vi "_LoadParameterTable.vi"(6 "ScanMode":string="Q1Pos") -> (0 "error out":errorcluster, 2 "ParameterList":string[][](array[string])=[["Q1 RF", "1", "10", "2150", "400", "0", "218.45", "64", "Quadrupole 1 RF", "\n      ", "\n      "], ["Q1 DC", "4", "10", "2150", "600", "0", "218.45", "64", "Quadrupole 1 DC", "\n      ", "\n      "], ["Q1 RR", "7", "0", "64000", "32768", "32768", "1", "64", "Quadrupole 1 PW", "\n      ", "\n      "], ["Q2 RF", "2", "10", "2150", "400", "0", "218.45", "64", "Quadrupole 2 RF", "\n      ", "\n      "], ["Q2 DC", "5", "10", "2150", "600", "0", "218.45", "64", "Quadrupole 2 DC", "\n      ", "\n      "], ["Q2 RR", "9", "0", "64000", "32768", "32768", "1", "64", "Quadrupole 2 PW", "\n      ", "\n      "], ["M1 RF", "3", "0", "600", "500", "0", "14.7", "6", "Multipole 1 RF", "Fixed", "Operator"], ["EV", "20", "0", "200", "100", "32768", "-65.7", "7", "Entrance Voltage", "Operator", "Operator"], ["ED", "21", "0", "200", "90", "32768", "-65.5", "7", "Entrance Deflector", "Operator", "Operator"], ["M1", "19", "-10", "5", "-1", "32768", "-65.6", "7", "Multipole 1", "Equation", "Equation"], ["L1", "18", "-10", "5", "-2", "32760", "-65.9", "7", "Multipole Lens 1", "Equation", "Equation"], ["M2", "22", "-10", "5", "-3", "32768", "-66", "7", "Multipole 2", "Fixed", "Fixed"], ["L2", "11", "-10", "5", "-4", "32768", "-65.9", "7", "Multipole Lens 2", "Equation", "Equation"], ["PF", "12", "-50", "5", "-15", "32768", "-65.8", "7", "Prefilter 1", "Equation", "Operator"], ["Q1", "6", "-10", "0", "-4.5", "32755", "-131.3", "11", "Quadrupole 1", "Equation", "Equation"], ["CC L1", "13", "-100", "10", "-10", "32768", "-65.8", "7", "Collision Cell Lens 1", "Equation", "Operator"], ["CC L2", "14", "-400", "0", "-120", "32768", "-65.8", "7", "Collision Cell Lens 2", "Fixed", "Operator"], ["CC", "23", "-150", "0", "-50", "32768", "-65.8", "7", "Collision Energy", "Fixed", "Fixed"], ["CC AF", "10", "0", "400", "100", "32768", "-65.8", "7", "Axial Field", "Fixed", "Fixed"], ["CC L3", "15", "-400", "0", "-51", "32768", "-65.7", "7", "Collision Cell Lens 3", "Equation", "Operator"], ["CC L4", "16", "-400", "0", "-62", "32768", "-65.7", "7", "Collision Cell Lens 4", "Equation", "Operator"], ["Q2", "8", "-150", "0", "-52", "32756", "-131.3", "11", "Quadrupole 2", "Equation", "Equation"], ["ID", "17", "-400", "0", "-90", "32768", "-65.8", "7", "Detector Deflector", "Equation", "Equation"], ["DISC", "32", "10", "2000", "15", "-5", "1.23", "18", "Discriminator", "Fixed", "Fixed"], ["DV", "34", "1600", "3500", "2000", "0", "0.415", "18", "Detector Voltage", "Operator", "Operator"], ["DET horn", "200", "0", "5500", "5500", "0", "0.415", "16", "Detector Horn", "Fixed", "Fixed"], ["LS400A", "36", "0", "420", "420", "0", "8.4", "64", "Lens Power Supply A +400", "\n      ", "\n      "], ["LS-400A", "37", "-420", "-55", "-420", "-433", "-8.4", "64", "Lens Power Supply A -400", "\n      ", "\n      "], ["LS400B", "38", "0", "420", "420", "0", "8.4", "64", "Lens Power Supply B +400", "\n      ", "\n      "], ["LS-400B", "39", "-420", "-55", "-420", "-433", "-8.4", "64", "Lens Power Supply B  -400", "\n      ", "\n      "], ["QPS800", "40", "110", "600", "600", "0", "4.25", "64", "Quad Power Supply +800", "\n      ", "\n      "], ["QPS-800", "41", "-110", "-110", "-600", "-433", "-4.2", "64", "Quad Power Supply -800", "\n      ", "\n      "], ["DG", "26", "50", "300", "80", "0", "32.765", "32", "Drying Gas", "Operator", "Operator"], ["NG1", "27", "0", "450", "0", "0", "32.765", "32", "Nebulizer Gas 1", "Operator", "Operator"], ["HG1", "29", "0", "350", "0", "0", "32.765", "32", "Heating Gas 1", "Equation", "Equation"], ["NG2", "28", "0", "450", "0", "0", "32.765", "32", "Nebulizer Gas 2", "Operator", "Operator"], ["HG2", "30", "0", "350", "0", "0", "32.765", "32", "Heating Gas 2", "Equation", "Equation"], ["CC P", "43", "0", "500", "0", "0", "32.765", "6", "Collision Pressure", "Fixed", "Fixed"], ["SX", "42", "0", "500", "500", "0", "32.765", "32", "Source Exhaust", "Fixed", "Fixed"], ["ISV2", "204", "0", "5850", "0", "0", "0.0436", "34", "ElectroSpray V2", "Operator", "Operator"], ["ISV1", "203", "0", "5850", "0", "0", "0.0436", "34", "ElectroSpray V1", "Operator", "Operator"], ["CD", "202", "0", "5", "0", "0", "51", "34", "Corona Discharge", "Operator", "Operator"], ["CAP", "201", "0", "1100", "1000", "0", "0.22", "34", "Curtain Cap", "Fixed", "Fixed"], ["HSID T", "81", "0", "320", "200", "0", "1", "32", "HSID Temperature", "Operator", "Operator"], ["P1 T", "86", "0", "500", "0", "0", "1", "32", "Source 1 Temp", "Operator", "Operator"], ["P2 T", "84", "0", "500", "0", "0", "1", "32", "Source 2 Temp", "Operator", "Operator"]])   [LabVIEW 2012]
uses:
  <vilib>/xml/Load XML File.vi
  <vilib>/xml/Close Reference(Node).vi
  <vilib>/xml/NI_XML.lvlib
  <resource>/objmgr/DOMUserDefRef.rc
panel:
  out "ScanType":string[](array[string])=["<ScanType name=\"Q1Positive\">\n    <ParaRow Row=\"1\">\n      <Parameter>Q1 RF</Parameter>\n      <Channal>1</Channal>\n      <UserMin>10</UserMin>\n      <UserMax>2150</UserMax>\n      <UserDefault>400</UserDefault>\n      <CalibrationOffset>0</CalibrationOffset>\n      <CalibrationSlope>218.45</CalibrationSlope>\n      <ParameterType>64</ParameterType>\n      <Description>Quadrupole 1 RF</Description>\n      <Linked>\n      </Linked>\n      <Unlinked>\n      </Unlinked>\n      <Location>\n      </Location>\n    </ParaRow>\n    <ParaRow Row=\"2\">\n      <Parameter>Q1 DC</Parameter>\n      <Channal>4</Channal>\n      <UserMin>10</UserMin>\n      <UserMax>2150</UserMax>\n      <UserDefault>600</UserDefault>\n      <CalibrationOffset>0</CalibrationOffset>\n      <CalibrationSlope>218.45</CalibrationSlope>\n      <ParameterType>64</ParameterType>\n      <Description>Quadrupole 1 DC</Description>\n      <Linked>\n      </Linked>\n      <Unlinked>\n      </Unlinked>\n      <Location>\n      </Location>\n    </ParaRow>\n    <ParaRow Row=\"3\">\n      <Parameter>Q1 RR</Parameter>\n      <Channal>7</Channal>\n      <UserMin>0</UserMin>\n      <UserMax>64000</UserMax>\n      <UserDefault>32768</UserDefault>\n      <CalibrationOffset>32768</CalibrationOffset>\n      <CalibrationSlope>1</CalibrationSlope>\n      <ParameterType>64</ParameterType>\n      <Description>Quadrupole 1 PW</Description>\n      <Linked>\n      </Linked>\n      <Unlinked>\n      </Unlinked>\n      <Location>\n      </Location>\n    </ParaRow>\n    <ParaRow Row=\"4\">\n      <Parameter>Q2 RF</Parameter>\n      <Channal>2</Channal>\n      <UserMin>10</UserMin>\n      <UserMax>2150</UserMax>\n      <UserDefault>400</UserDefault>\n      <CalibrationOffset>0</CalibrationOffset>\n      <CalibrationSlope>218.45</CalibrationSlope>\n      <ParameterType>64</ParameterType>\n      <Description>Quadrupole 2 RF</Description>\n      <Linked>\n      </Linked>\n      <Unlinked>\n      </Unlinked>\n      <Location>\n      </Location>\n    </ParaRow>\n    <ParaRow Row=\"5\">\n      <Parameter>Q2 DC</Parameter>\n      <Channal>5</Channal>\n      <UserMin>10</UserMin>\n      <UserMax>2150</UserMax>\n      <UserDefault>600</UserDefault>\n      <CalibrationOffset>0</CalibrationOffset>\n      <CalibrationSlope>218.45</CalibrationSlope>\n      <ParameterType>64</ParameterType>\n      <Description>Quadrupole 2 DC</Description>\n      <Linked>\n      </Linked>\n      <Unlinked>\n      </Unlinked>\n      <Location>\n      </Location>\n    </ParaRow>\n    <ParaRow Row=\"6\">\n      <Parameter>Q2 RR</Parameter>\n      <Channal>9</Channal>\n      <UserMin>0</UserMin>\n      <UserMax>64000</UserMax>\n      <UserDefault>32768</UserDefault>\n      <CalibrationOffset>32768</CalibrationOffset>\n      <CalibrationSlope>1</CalibrationSlope>\n      <ParameterType>64</ParameterType>\n      <Description>Quadrupole 2 PW</Description>\n      <Linked>\n      </Linked>\n      <Unlinked>\n      </Unlinked>\n      <Location>\n      </Location>\n    </ParaRow>\n    <ParaRow Row=\"7\">\n      <Parameter>M1 RF</Parameter>\n      <Channal>3</Channal>\n      <UserMin>0</UserMin>\n      <UserMax>600</UserMax>\n      <UserDefault>500</UserDefault>\n      <CalibrationOffset>0</CalibrationOffset>\n      <CalibrationSlope>14.7</CalibrationSlope>\n      <ParameterType>6</ParameterType>\n      <Description>Multipole 1 RF</Description>\n      <Linked>Fixed</Linked>\n      <Unlinked>Operator</Unlinked>\n      <Location>Compound</Location>\n    </ParaRow>\n    <ParaRow Row=\"8\">\n      <Parameter>EV</Parameter>\n      <Channal>20</Channal>\n      <UserMin>0</UserMin>\n      <UserMax>200</UserMax>\n      <UserDefault>100</UserDefault>\n      <CalibrationOffset>32768</CalibrationOffset>\n      <CalibrationSlope>-65.7</CalibrationSlope>\n      <ParameterType>7</ParameterType>\n      <Description>Entrance Voltage</Description>\n      <Linked>Operator</Linked>\n      <Unlinked>Operator</Unlinked>\n      <Location>Compound</Location>\n    </ParaRow>\n    <ParaRow Row=\"9\">\n      <Parameter>ED</Parameter>\n      <Channal>21</Channal>\n      <UserMin>0</UserMin>\n      <UserMax>200</UserMax>\n      <UserDefault>90</UserDefault>\n      <CalibrationOffset>32768</CalibrationOffset>\n      <CalibrationSlope>-65.5</CalibrationSlope>\n      <ParameterType>7</ParameterType>\n      <Description>Entrance Deflector</Description>\n      <Linked>Operator</Linked>\n      <Unlinked>Operator</Unlinked>\n      <Location>Compound</Location>\n    </ParaRow>\n    <ParaRow Row=\"10\">\n      <Parameter>M1</Parameter>\n      <Channal>19</Channal>\n      <UserMin>-10</UserMin>\n      <UserMax>5</UserMax>\n      <UserDefault>-1</UserDefault>\n      <CalibrationOffset>32768</CalibrationOffset>\n      <CalibrationSlope>-65.6</CalibrationSlope>\n      <ParameterType>7</ParameterType>\n      <Description>Multipole 1</Description>\n      <Linked>Equation</Linked>\n      <Unlinked>Equation</Unlinked>\n      <Location>Compound</Location>\n    </ParaRow>\n    <ParaRow Row=\"11\">\n      <Parameter>L1</Parameter>\n      <Channal>18</Channal>\n      <UserMin>-10</UserMin>\n      <UserMax>5</UserMax>\n      <UserDefault>-2</UserDefault>\n      <CalibrationOffset>32760</CalibrationOffset>\n      <CalibrationSlope>-65.9</CalibrationSlope>\n      <ParameterType>7</ParameterType>\n      <Description>Multipole Lens 1</Description>\n      <Linked>Equation</Linked>\n      <Unlinked>Equation</Unlinked>\n      <Location>Compound</Location>\n    </ParaRow>\n    <ParaRow Row=\"12\">\n      <Parameter>M2</Parameter>\n      <Channal>22</Channal>\n      <UserMin>-10</UserMin>\n      <UserMax>5</UserMax>\n      <UserDefault>-3</UserDefault>\n      <CalibrationOffset>32768</CalibrationOffset>\n      <CalibrationSlope>-66</CalibrationSlope>\n      <ParameterType>7</ParameterType>\n      <Description>Multipole 2</Description>\n      <Linked>Fixed</Linked>\n      <Unlinked>Fixed</Unlinked>\n      <Location>Compound</Location>\n    </ParaRow>\n    <ParaRow Row=\"13\">\n      <Parameter>L2</Parameter>\n      <Channal>11</Channal>\n      <UserMin>-10</UserMin>\n      <UserMax>5</UserMax>\n      <UserDefault>-4</UserDefault>\n      <CalibrationOffset>32768</CalibrationOffset>\n      <CalibrationSlope>-65.9</CalibrationSlope>\n      <ParameterType>7</ParameterType>\n      <Description>Multipole Lens 2</Description>\n      <Linked>Equation</Linked>\n      <Unlinked>Equation</Unlinked>\n      <Location>Compound</Location>\n    </ParaRow>\n    <ParaRow Row=\"14\">\n      <Parameter>PF</Parameter>\n      <Channal>12</Channal>\n      <UserMin>-50</UserMin>\n      <UserMax>5</UserMax>\n      <UserDefault>-15</UserDefault>\n      <CalibrationOffset>32768</CalibrationOffset>\n      <CalibrationSlope>-65.8</CalibrationSlope>\n      <ParameterType>7</ParameterType>\n      <Description>Prefilter 1</Description>\n      <Linked>Equation</Linked>\n      <Unlinked>Operator</Unlinked>\n      <Location>Compound</Location>\n    </ParaRow>\n    <ParaRow Row=\"15\">\n      <Parameter>Q1</Parameter>\n      <Channal>6</Channal>\n      <UserMin>-10</UserMin>\n      <UserMax>0</UserMax>\n      <UserDefault>-4.5</UserDefault>\n      <CalibrationOffset>32755</CalibrationOffset>\n      <CalibrationSlope>-131.3</CalibrationSlope>\n      <ParameterType>11</ParameterType>\n      <Description>Quadrupole 1</Description>\n      <Linked>Equation</Linked>\n      <Unlinked>Equation</Unlinked>\n      <Location>Resolution</Location>\n    </ParaRow>\n    <ParaRow Row=\"16\">\n      <Parameter>CC L1</Parameter>\n      <Channal>13</Channal>\n      <UserMin>-100</UserMin>\n      <UserMax>10</UserMax>\n      <UserDefault>-10</UserDefault>\n      <CalibrationOffset>32768</CalibrationOffset>\n      <CalibrationSlope>-65.8</CalibrationSlope>\n      <ParameterType>7</ParameterType>\n      <Description>Collision Cell Lens 1</Description>\n      <Linked>Equation</Linked>\n      <Unlinked>Operator</Unlinked>\n      <Location>Compound</Location>\n    </ParaRow>\n    <ParaRow Row=\"17\">\n      <Parameter>CC L2</Parameter>\n      <Channal>14</Channal>\n      <UserMin>-400</UserMin>\n      <UserMax>0</UserMax>\n      <UserDefault>-120</UserDefault>\n      <CalibrationOffset>32768</CalibrationOffset>\n      <CalibrationSlope>-65.8</CalibrationSlope>\n      <ParameterType>7</ParameterType>\n      <Description>Collision Cell Lens 2</Description>\n      <Linked>Fixed</Linked>\n      <Unlinked>Operator</Unlinked>\n      <Location>Compound</Location>\n    </ParaRow>\n    <ParaRow Row=\"18\">\n      <Parameter>CC</Parameter>\n      <Channal>23</Channal>\n      <UserMin>-150</UserMin>\n      <UserMax>0</UserMax>\n      <UserDefault>-50</UserDefault>\n      <CalibrationOffset>32768</CalibrationOffset>\n      <CalibrationSlope>-65.8</CalibrationSlope>\n      <ParameterType>7</ParameterType>\n      <Description>Collision Energy</Description>\n      <Linked>Fixed</Linked>\n      <Unlinked>Fixed</Unlinked>\n      <Location>Compound</Location>\n    </ParaRow>\n    <ParaRow Row=\"19\">\n      <Parameter>CC AF</Parameter>\n      <Channal>10</Channal>\n      <UserMin>0</UserMin>\n      <UserMax>400</UserMax>\n      <UserDefault>100</UserDefault>\n      <CalibrationOffset>32768</CalibrationOffset>\n      <CalibrationSlope>-65.8</CalibrationSlope>\n      <ParameterType>7</ParameterType>\n      <Description>Axial Field</Description>\n      <Linked>Fixed</Linked>\n      <Unlinked>Fixed</Unlinked>\n      <Location>Compound</Location>\n    </ParaRow>\n    <ParaRow Row=\"20\">\n      <Parameter>CC L3</Parameter>\n      <Channal>15</Channal>\n      <UserMin>-400</UserMin>\n      <UserMax>0</UserMax>\n      <UserDefault>-51</UserDefault>\n      <CalibrationOffset>32768</CalibrationOffset>\n      <CalibrationSlope>-65.7</CalibrationSlope>\n      <ParameterType>7</ParameterType>\n      <Description>Collision Cell Lens 3</Description>\n      <Linked>Equation</Linked>\n      <Unlinked>Operator</Unlinked>\n      <Location>Compound</Location>\n    </ParaRow>\n    <ParaRow Row=\"21\">\n      <Parameter>CC L4</Parameter>\n      <Channal>16</Channal>\n      <UserMin>-400</UserMin>\n      <UserMax>0</UserMax>\n      <UserDefault>-62</UserDefault>\n      <CalibrationOffset>32768</CalibrationOffset>\n      <CalibrationSlope>-65.7</CalibrationSlope>\n      <ParameterType>7</ParameterType>\n      <Description>Collision Cell Lens 4</Description>\n      <Linked>Equation</Linked>\n      <Unlinked>Operator</Unlinked>\n      <Location>Compound</Location>\n    </ParaRow>\n    <ParaRow Row=\"22\">\n      <Parameter>Q2</Parameter>\n      <Channal>8</Channal>\n      <UserMin>-150</UserMin>\n      <UserMax>0</UserMax>\n      <UserDefault>-52</UserDefault>\n      <CalibrationOffset>32756</CalibrationOffset>\n      <CalibrationSlope>-131.3</CalibrationSlope>\n      <ParameterType>11</ParameterType>\n      <Description>Quadrupole 2</Description>\n      <Linked>Equation</Linked>\n      <Unlinked>Equation</Unlinked>\n      <Location>Resolution</Location>\n    </ParaRow>\n    <ParaRow Row=\"23\">\n      <Parameter>ID</Parameter>\n      <Channal>17</Channal>\n      <UserMin>-400</UserMin>\n      <UserMax>0</UserMax>\n      <UserDefault>-90</UserDefault>\n      <CalibrationOffset>32768</CalibrationOffset>\n      <CalibrationSlope>-65.8</CalibrationSlope>\n      <ParameterType>7</ParameterType>\n      <Description>Detector Deflector</Description>\n      <Linked>Equation</Linked>\n      <Unlinked>Equation</Unlinked>\n      <Location>Compound</Location>\n    </ParaRow>\n    <ParaRow Row=\"24\">\n      <Parameter>DISC</Parameter>\n      <Channal>32</Channal>\n      <UserMin>10</UserMin>\n      <UserMax>2000</UserMax>\n      <UserDefault>15</UserDefault>\n      <CalibrationOffset>-5</CalibrationOffset>\n      <CalibrationSlope>1.23</CalibrationSlope>\n      <ParameterType>18</ParameterType>\n      <Description>Discriminator</Description>\n      <Linked>Fixed</Linked>\n      <Unlinked>Fixed</Unlinked>\n      <Location>Detector</Location>\n    </ParaRow>\n    <ParaRow Row=\"25\">\n      <Parameter>DV</Parameter>\n      <Channal>34</Channal>\n      <UserMin>1600</UserMin>\n      <UserMax>3500</UserMax>\n      <UserDefault>2000</UserDefault>\n      <CalibrationOffset>0</CalibrationOffset>\n      <CalibrationSlope>0.415</CalibrationSlope>\n      <ParameterType>18</ParameterType>\n      <Description>Detector Voltage</Description>\n      <Linked>Operator</Linked>\n      <Unlinked>Operator</Unlinked>\n      <Location>Detector</Location>\n    </ParaRow>\n    <ParaRow Row=\"26\">\n      <Parameter>DET horn</Parameter>\n      <Channal>200</Channal>\n      <UserMin>0</UserMin>\n      <UserMax>5500</UserMax>\n      <UserDefault>5500</UserDefault>\n      <CalibrationOffset>0</CalibrationOffset>\n      <CalibrationSlope>0.415</CalibrationSlope>\n      <ParameterType>16</ParameterType>\n      <Description>Detector Horn</Description>\n      <Linked>Fixed</Linked>\n      <Unlinked>Fixed</Unlinked>\n      <Location>Detector</Location>\n    </ParaRow>\n    <ParaRow Row=\"27\">\n      <Parameter>LS400A</Parameter>\n      <Channal>36</Channal>\n      <UserMin>0</UserMin>\n      <UserMax>420</UserMax>\n      <UserDefault>420</UserDefault>\n      <CalibrationOffset>0</CalibrationOffset>\n      <CalibrationSlope>8.4</CalibrationSlope>\n      <ParameterType>64</ParameterType>\n      <Description>Lens Power Supply A +400</Description>\n      <Linked>\n      </Linked>\n      <Unlinked>\n      </Unlinked>\n      <Location>\n      </Location>\n    </ParaRow>\n    <ParaRow Row=\"28\">\n      <Parameter>LS-400A</Parameter>\n      <Channal>37</Channal>\n      <UserMin>-420</UserMin>\n      <UserMax>-55</UserMax>\n      <UserDefault>-420</UserDefault>\n      <CalibrationOffset>-433</CalibrationOffset>\n      <CalibrationSlope>-8.4</CalibrationSlope>\n      <ParameterType>64</ParameterType>\n      <Description>Lens Power Supply A -400</Description>\n      <Linked>\n      </Linked>\n      <Unlinked>\n      </Unlinked>\n      <Location>\n      </Location>\n    </ParaRow>\n    <ParaRow Row=\"29\">\n      <Parameter>LS400B</Parameter>\n      <Channal>38</Channal>\n      <UserMin>0</UserMin>\n      <UserMax>420</UserMax>\n      <UserDefault>420</UserDefault>\n      <CalibrationOffset>0</CalibrationOffset>\n      <CalibrationSlope>8.4</CalibrationSlope>\n      <ParameterType>64</ParameterType>\n      <Description>Lens Power Supply B +400</Description>\n      <Linked>\n      </Linked>\n      <Unlinked>\n      </Unlinked>\n      <Location>\n      </Location>\n    </ParaRow>\n    <ParaRow Row=\"30\">\n      <Parameter>LS-400B</Parameter>\n      <Channal>39</Channal>\n      <UserMin>-420</UserMin>\n      <UserMax>-55</UserMax>\n      <UserDefault>-420</UserDefault>\n      <CalibrationOffset>-433</CalibrationOffset>\n      <CalibrationSlope>-8.4</CalibrationSlope>\n      <ParameterType>64</ParameterType>\n      <Description>Lens Power Supply B  -400</Description>\n      <Linked>\n      </Linked>\n      <Unlinked>\n      </Unlinked>\n      <Location>\n      </Location>\n    </ParaRow>\n    <ParaRow Row=\"31\">\n      <Parameter>QPS800</Parameter>\n      <Channal>40</Channal>\n      <UserMin>110</UserMin>\n      <UserMax>600</UserMax>\n      <UserDefault>600</UserDefault>\n      <CalibrationOffset>0</CalibrationOffset>\n      <CalibrationSlope>4.25</CalibrationSlope>\n      <ParameterType>64</ParameterType>\n      <Description>Quad Power Supply +800</Description>\n      <Linked>\n      </Linked>\n      <Unlinked>\n      </Unlinked>\n      <Location>\n      </Location>\n    </ParaRow>\n    <ParaRow Row=\"32\">\n      <Parameter>QPS-800</Parameter>\n      <Channal>41</Channal>\n      <UserMin>-110</UserMin>\n      <UserMax>-110</UserMax>\n      <UserDefault>-600</UserDefault>\n      <CalibrationOffset>-433</CalibrationOffset>\n      <CalibrationSlope>-4.2</CalibrationSlope>\n      <ParameterType>64</ParameterType>\n      <Description>Quad Power Supply -800</Description>\n      <Linked>\n      </Linked>\n      <Unlinked>\n      </Unlinked>\n      <Location>\n      </Location>\n    </ParaRow>\n    <ParaRow Row=\"33\">\n      <Parameter>DG</Parameter>\n      <Channal>26</Channal>\n      <UserMin>50</UserMin>\n      <UserMax>300</UserMax>\n      <UserDefault>80</UserDefault>\n      <CalibrationOffset>0</CalibrationOffset>\n      <CalibrationSlope>32.765</CalibrationSlope>\n      <ParameterType>32</ParameterType>\n      <Description>Drying Gas</Description>\n      <Linked>Operator</Linked>\n      <Unlinked>Operator</Unlinked>\n      <Location>Source</Location>\n    </ParaRow>\n    <ParaRow Row=\"34\">\n      <Parameter>NG1</Parameter>\n      <Channal>27</Channal>\n      <UserMin>0</UserMin>\n      <UserMax>450</UserMax>\n      <UserDefault>0</UserDefault>\n      <CalibrationOffset>0</CalibrationOffset>\n      <CalibrationSlope>32.765</CalibrationSlope>\n      <ParameterType>32</ParameterType>\n      <Description>Nebulizer Gas 1</Description>\n      <Linked>Operator</Linked>\n      <Unlinked>Operator</Unlinked>\n      <Location>Source</Location>\n    </ParaRow>\n    <ParaRow Row=\"35\">\n      <Parameter>HG1</Parameter>\n      <Channal>29</Channal>\n      <UserMin>0</UserMin>\n      <UserMax>350</UserMax>\n      <UserDefault>0</UserDefault>\n      <CalibrationOffset>0</CalibrationOffset>\n      <CalibrationSlope>32.765</CalibrationSlope>\n      <ParameterType>32</ParameterType>\n      <Description>Heating Gas 1</Description>\n      <Linked>Equation</Linked>\n      <Unlinked>Equation</Unlinked>\n      <Location>Source</Location>\n    </ParaRow>\n    <ParaRow Row=\"36\">\n      <Parameter>NG2</Parameter>\n      <Channal>28</Channal>\n      <UserMin>0</UserMin>\n      <UserMax>450</UserMax>\n      <UserDefault>0</UserDefault>\n      <CalibrationOffset>0</CalibrationOffset>\n      <CalibrationSlope>32.765</CalibrationSlope>\n      <ParameterType>32</ParameterType>\n      <Description>Nebulizer Gas 2</Description>\n      <Linked>Operator</Linked>\n      <Unlinked>Operator</Unlinked>\n      <Location>Source</Location>\n    </ParaRow>\n    <ParaRow Row=\"37\">\n      <Parameter>HG2</Parameter>\n      <Channal>30</Channal>\n      <UserMin>0</UserMin>\n      <UserMax>350</UserMax>\n      <UserDefault>0</UserDefault>\n      <CalibrationOffset>0</CalibrationOffset>\n      <CalibrationSlope>32.765</CalibrationSlope>\n      <ParameterType>32</ParameterType>\n      <Description>Heating Gas 2</Description>\n      <Linked>Equation</Linked>\n      <Unlinked>Equation</Unlinked>\n      <Location>Source</Location>\n    </ParaRow>\n    <ParaRow Row=\"38\">\n      <Parameter>CC P</Parameter>\n      <Channal>43</Channal>\n      <UserMin>0</UserMin>\n      <UserMax>500</UserMax>\n      <UserDefault>0</UserDefault>\n      <CalibrationOffset>0</CalibrationOffset>\n      <CalibrationSlope>32.765</CalibrationSlope>\n      <ParameterType>6</ParameterType>\n      <Description>Collision Pressure</Description>\n      <Linked>Fixed</Linked>\n      <Unlinked>Fixed</Unlinked>\n      <Location>Compound</Location>\n    </ParaRow>\n    <ParaRow Row=\"39\">\n      <Parameter>SX</Parameter>\n      <Channal>42</Channal>\n      <UserMin>0</UserMin>\n      <UserMax>500</UserMax>\n      <UserDefault>500</UserDefault>\n      <CalibrationOffset>0</CalibrationOffset>\n      <CalibrationSlope>32.765</CalibrationSlope>\n      <ParameterType>32</ParameterType>\n      <Description>Source Exhaust</Description>\n      <Linked>Fixed</Linked>\n      <Unlinked>Fixed</Unlinked>\n      <Location>Source</Location>\n    </ParaRow>\n    <ParaRow Row=\"40\">\n      <Parameter>ISV2</Parameter>\n      <Channal>204</Channal>\n      <UserMin>0</UserMin>\n      <UserMax>5850</UserMax>\n      <UserDefault>0</UserDefault>\n      <CalibrationOffset>0</CalibrationOffset>\n      <CalibrationSlope>0.0436</CalibrationSlope>\n      <ParameterType>34</ParameterType>\n      <Description>ElectroSpray V2</Description>\n      <Linked>Operator</Linked>\n      <Unlinked>Operator</Unlinked>\n      <Location>Source</Location>\n    </ParaRow>\n    <ParaRow Row=\"41\">\n      <Parameter>ISV1</Parameter>\n      <Channal>203</Channal>\n      <UserMin>0</UserMin>\n      <UserMax>5850</UserMax>\n      <UserDefault>0</UserDefault>\n      <CalibrationOffset>0</CalibrationOffset>\n      <CalibrationSlope>0.0436</CalibrationSlope>\n      <ParameterType>34</ParameterType>\n      <Description>ElectroSpray V1</Description>\n      <Linked>Operator</Linked>\n      <Unlinked>Operator</Unlinked>\n      <Location>Source</Location>\n    </ParaRow>\n    <ParaRow Row=\"42\">\n      <Parameter>CD</Parameter>\n      <Channal>202</Channal>\n      <UserMin>0</UserMin>\n      <UserMax>5</UserMax>\n      <UserDefault>0</UserDefault>\n      <CalibrationOffset>0</CalibrationOffset>\n      <CalibrationSlope>51</CalibrationSlope>\n      <ParameterType>34</ParameterType>\n      <Description>Corona Discharge</Description>\n      <Linked>Operator</Linked>\n      <Unlinked>Operator</Unlinked>\n      <Location>Source</Location>\n    </ParaRow>\n    <ParaRow Row=\"43\">\n      <Parameter>CAP</Parameter>\n      <Channal>201</Channal>\n      <UserMin>0</UserMin>\n      <UserMax>1100</UserMax>\n      <UserDefault>1000</UserDefault>\n      <CalibrationOffset>0</CalibrationOffset>\n      <CalibrationSlope>0.22</CalibrationSlope>\n      <ParameterType>34</ParameterType>\n      <Description>Curtain Cap</Description>\n      <Linked>Fixed</Linked>\n      <Unlinked>Fixed</Unlinked>\n      <Location>Source</Location>\n    </ParaRow>\n    <ParaRow Row=\"44\">\n      <Parameter>HSID T</Parameter>\n      <Channal>81</Channal>\n      <UserMin>0</UserMin>\n      <UserMax>320</UserMax>\n      <UserDefault>200</UserDefault>\n      <CalibrationOffset>0</CalibrationOffset>\n      <CalibrationSlope>1</CalibrationSlope>\n      <ParameterType>32</ParameterType>\n      <Description>HSID Temperature</Description>\n      <Linked>Operator</Linked>\n      <Unlinked>Operator</Unlinked>\n      <Location>Source</Location>\n    </ParaRow>\n    <ParaRow Row=\"45\">\n      <Parameter>P1 T</Parameter>\n      <Channal>86</Channal>\n      <UserMin>0</UserMin>\n      <UserMax>500</UserMax>\n      <UserDefault>0</UserDefault>\n      <CalibrationOffset>0</CalibrationOffset>\n      <CalibrationSlope>1</CalibrationSlope>\n      <ParameterType>32</ParameterType>\n      <Description>Source 1 Temp</Description>\n      <Linked>Operator</Linked>\n      <Unlinked>Operator</Unlinked>\n      <Location>Source</Location>\n    </ParaRow>\n    <ParaRow Row=\"46\">\n      <Parameter>P2 T</Parameter>\n      <Channal>84</Channal>\n      <UserMin>0</UserMin>\n      <UserMax>500</UserMax>\n      <UserDefault>0</UserDefault>\n      <CalibrationOffset>0</CalibrationOffset>\n      <CalibrationSlope>1</CalibrationSlope>\n      <ParameterType>32</ParameterType>\n      <Description>Source 2 Temp</Description>\n      <Linked>Operator</Linked>\n      <Unlinked>Operator</Unlinked>\n      <Location>Source</Location>\n    </ParaRow>\n  </ScanType>", "<ScanType name=\"Q1Negative\">\n    <ParaRow Row=\"1\">\n      <Parameter>Q1 RF</Parameter>\n      <Channal>1</Channal>\n      <UserMin>10</UserMin>\n      <UserMax>2150</UserMax>\n      <UserDefault>400</UserDefault>\n      <CalibrationOffset>0</CalibrationOffset>\n      <CalibrationSlope>218.45</CalibrationSlope>\n      <ParameterType>64</ParameterType>\n      <Description>Quadrupole 1 RF</Description>\n      <Linked>\n      </Linked>\n      <Unlinked>\n      </Unlinked>\n      <Location>\n      </Location>\n    </ParaRow>\n    <ParaRow Row=\"2\">\n      <Parameter>Q1 DC</Parameter>\n      <Channal>4</Channal>\n      <UserMin>10</UserMin>\n      <UserMax>2150</UserMax>\n      <UserDefault>600</UserDefault>\n      <CalibrationOffset>0</CalibrationOffset>\n      <CalibrationSlope>218.45</CalibrationSlope>\n      <ParameterType>64</ParameterType>\n      <Description>Quadrupole 1 DC</Description>\n      <Linked>\n      </Linked>\n      <Unlinked>\n      </Unlinked>\n      <Location>\n      </Location>\n    </ParaRow>\n    <ParaRow Row=\"3\">\n      <Parameter>Q1 RR</Parameter>\n      <Channal>7</Channal>\n      <UserMin>0</UserMin>\n      <UserMax>64000</UserMax>\n      <UserDefault>32768</UserDefault>\n      <CalibrationOffset>32768</CalibrationOffset>\n      <CalibrationSlope>1</CalibrationSlope>\n      <ParameterType>64</ParameterType>\n      <Description>Quadrupole 1 PW</Description>\n      <Linked>\n      </Linked>\n      <Unlinked>\n      </Unlinked>\n      <Location>\n      </Location>\n    </ParaRow>\n    <ParaRow Row=\"4\">\n      <Parameter>Q2 RF</Parameter>\n      <Channal>2</Channal>\n      <UserMin>10</UserMin>\n      <UserMax>2150</UserMax>\n      <UserDefault>400</UserDefault>\n      <CalibrationOffset>0</CalibrationOffset>\n      <CalibrationSlope>218.45</CalibrationSlope>\n      <ParameterType>64</ParameterType>\n      <Description>Quadrupole 2 RF</Description>\n      <Linked>\n      </Linked>\n      <Unlinked>\n      </Unlinked>\n      <Location>\n      </Location>\n    </ParaRow>\n    <ParaRow Row=\"5\">\n      <Parameter>Q2 DC</Parameter>\n      <Channal>5</Channal>\n      <UserMin>10</UserMin>\n      <UserMax>2150</UserMax>\n      <UserDefault>600</UserDefault>\n      <CalibrationOffset>0</CalibrationOffset>\n      <CalibrationSlope>218.45</CalibrationSlope>\n      <ParameterType>64</ParameterType>\n      <Description>Quadrupole 2 DC</Description>\n      <Linked>\n      </Linked>\n      <Unlinked>\n      </Unlinked>\n      <Location>\n      </Location>\n    </ParaRow>\n    <ParaRow Row=\"6\">\n      <Parameter>Q2 RR</Parameter>\n      <Channal>9</Channal>\n      <UserMin>0</UserMin>\n      <UserMax>64000</UserMax>\n      <UserDefault>32768</UserDefault>\n      <CalibrationOffset>32768</CalibrationOffset>\n      <CalibrationSlope>1</CalibrationSlope>\n      <ParameterType>64</ParameterType>\n      <Description>Quadrupole 2 PW</Description>\n      <Linked>\n      </Linked>\n      <Unlinked>\n      </Unlinked>\n      <Location>\n      </Location>\n    </ParaRow>\n    <ParaRow Row=\"7\">\n      <Parameter>M1 RF</Parameter>\n      <Channal>3</Channal>\n      <UserMin>0</UserMin>\n      <UserMax>600</UserMax>\n      <UserDefault>500</UserDefault>\n      <CalibrationOffset>0</CalibrationOffset>\n      <CalibrationSlope>14.7</CalibrationSlope>\n      <ParameterType>6</ParameterType>\n      <Description>Multipole 1 RF</Description>\n      <Linked>Fixed</Linked>\n      <Unlinked>Operator</Unlinked>\n      <Location>Compound</Location>\n    </ParaRow>\n    <ParaRow Row=\"8\">\n      <Parameter>EV</Parameter>\n      <Channal>20</Channal>\n      <UserMin>-200</UserMin>\n      <UserMax>0</UserMax>\n      <UserDefault>-100</UserDefault>\n      <CalibrationOffset>32768</CalibrationOffset>\n      <CalibrationSlope>-65.7</CalibrationSlope>\n      <ParameterType>7</ParameterType>\n      <Description>Entrance Voltage</Description>\n      <Linked>Operator</Linked>\n      <Unlinked>Operator</Unlinked>\n      <Location>Compound</Location>\n    </ParaRow>\n    <ParaRow Row=\"9\">\n      <Parameter>ED</Parameter>\n      <Channal>21</Channal>\n      <UserMin>-200</UserMin>\n      <UserMax>0</UserMax>\n      <UserDefault>-90</UserDefault>\n      <CalibrationOffset>32768</CalibrationOffset>\n      <CalibrationSlope>-65.5</CalibrationSlope>\n      <ParameterType>7</ParameterType>\n      <Description>Entrance Deflector</Description>\n      <Linked>Operator</Linked>\n      <Unlinked>Operator</Unlinked>\n      <Location>Compound</Location>\n    </ParaRow>\n    <ParaRow Row=\"10\">\n      <Parameter>M1</Parameter>\n      <Channal>19</Channal>\n      <UserMin>-5</UserMin>\n      <UserMax>10</UserMax>\n      <UserDefault>1</UserDefault>\n      <CalibrationOffset>32768</CalibrationOffset>\n      <CalibrationSlope>-65.6</CalibrationSlope>\n      <ParameterType>7</ParameterType>\n      <Description>Multipole 1</Description>\n      <Linked>Equation</Linked>\n      <Unlinked>Equation</Unlinked>\n      <Location>Compound</Location>\n    </ParaRow>\n    <ParaRow Row=\"11\">\n      <Parameter>L1</Parameter>\n      <Channal>18</Channal>\n      <UserMin>-5</UserMin>\n      <UserMax>10</UserMax>\n      <UserDefault>2</UserDefault>\n      <CalibrationOffset>32760</CalibrationOffset>\n      <CalibrationSlope>-65.9</CalibrationSlope>\n      <ParameterType>7</ParameterType>\n      <Description>Multipole Lens 1</Description>\n      <Linked>Equation</Linked>\n      <Unlinked>Equation</Unlinked>\n      <Location>Compound</Location>\n    </ParaRow>\n    <ParaRow Row=\"12\">\n      <Parameter>M2</Parameter>\n      <Channal>22</Channal>\n      <UserMin>-5</UserMin>\n      <UserMax>10</UserMax>\n      <UserDefault>3</UserDefault>\n      <CalibrationOffset>32768</CalibrationOffset>\n      <CalibrationSlope>-66</CalibrationSlope>\n      <ParameterType>7</ParameterType>\n      <Description>Multipole 2</Description>\n      <Linked>Fixed</Linked>\n      <Unlinked>Fixed</Unlinked>\n      <Location>Compound</Location>\n    </ParaRow>\n    <ParaRow Row=\"13\">\n      <Parameter>L2</Parameter>\n      <Channal>11</Channal>\n      <UserMin>-5</UserMin>\n      <UserMax>10</UserMax>\n      <UserDefault>4</UserDefault>\n      <CalibrationOffset>32768</CalibrationOffset>\n      <CalibrationSlope>-65.9</CalibrationSlope>\n      <ParameterType>7</ParameterType>\n      <Description>Multipole Lens 2</Description>\n      <Linked>Equation</Linked>\n      <Unlinked>Equation</Unlinked>\n      <Location>Compound</Location>\n    </ParaRow>\n    <ParaRow Row=\"14\">\n      <Parameter>PF</Parameter>\n      <Channal>12</Channal>\n      <UserMin>-5</UserMin>\n      <UserMax>50</UserMax>\n      <UserDefault>15</UserDefault>\n      <CalibrationOffset>32768</CalibrationOffset>\n      <CalibrationSlope>-65.8</CalibrationSlope>\n      <ParameterType>7</ParameterType>\n      <Description>Prefilter 1</Description>\n      <Linked>Equation</Linked>\n      <Unlinked>Operator</Unlinked>\n      <Location>Compound</Location>\n    </ParaRow>\n    <ParaRow Row=\"15\">\n      <Parameter>Q1</Parameter>\n      <Channal>6</Channal>\n      <UserMin>0</UserMin>\n      <UserMax>10</UserMax>\n      <UserDefault>4.5</UserDefault>\n      <CalibrationOffset>32755</CalibrationOffset>\n      <CalibrationSlope>-131.3</CalibrationSlope>\n      <ParameterType>11</ParameterType>\n      <Description>Quadrupole 1</Description>\n      <Linked>Equation</Linked>\n      <Unlinked>Equation</Unlinked>\n      <Location>Resolution</Location>\n    </ParaRow>\n    <ParaRow Row=\"16\">\n      <Parameter>CC L1</Parameter>\n      <Channal>13</Channal>\n      <UserMin>-10</UserMin>\n      <UserMax>100</UserMax>\n      <UserDefault>10</UserDefault>\n      <CalibrationOffset>32768</CalibrationOffset>\n      <CalibrationSlope>-65.8</CalibrationSlope>\n      <ParameterType>7</ParameterType>\n      <Description>Collision Cell Lens 1</Description>\n      <Linked>Equation</Linked>\n      <Unlinked>Operator</Unlinked>\n      <Location>Compound</Location>\n    </ParaRow>\n    <ParaRow Row=\"17\">\n      <Parameter>CC L2</Parameter>\n      <Channal>14</Channal>\n      <UserMin>0</UserMin>\n      <UserMax>400</UserMax>\n      <UserDefault>120</UserDefault>\n      <CalibrationOffset>32768</CalibrationOffset>\n      <CalibrationSlope>-65.8</CalibrationSlope>\n      <ParameterType>7</ParameterType>\n      <Description>Collision Cell Lens 2</Description>\n      <Linked>Fixed</Linked>\n      <Unlinked>Operator</Unlinked>\n      <Location>Compound</Location>\n    </ParaRow>\n    <ParaRow Row=\"18\">\n      <Parameter>CC</Parameter>\n      <Channal>23</Channal>\n      <UserMin>0</UserMin>\n      <UserMax>150</UserMax>\n      <UserDefault>50</UserDefault>\n      <CalibrationOffset>32768</CalibrationOffset>\n      <CalibrationSlope>-65.8</CalibrationSlope>\n      <ParameterType>7</ParameterType>\n      <Description>Collision Energy</Description>\n      <Linked>Fixed</Linked>\n      <Unlinked>Fixed</Unlinked>\n      <Location>Compound</Location>\n    </ParaRow>\n    <ParaRow Row=\"19\">\n      <Parameter>CC AF</Parameter>\n      <Channal>10</Channal>\n      <UserMin>-400</UserMin>\n      <UserMax>0</UserMax>\n      <UserDefault>-100</UserDefault>\n      <CalibrationOffset>32768</CalibrationOffset>\n      <CalibrationSlope>-65.8</CalibrationSlope>\n      <ParameterType>7</ParameterType>\n      <Description>Axial Field</Description>\n      <Linked>Fixed</Linked>\n      <Unlinked>Fixed</Unlinked>\n      <Location>Compound</Location>\n    </ParaRow>\n    <ParaRow Row=\"20\">\n      <Parameter>CC L3</Parameter>\n      <Channal>15</Channal>\n      <UserMin>0</UserMin>\n      <UserMax>400</UserMax>\n      <UserDefault>51</UserDefault>\n      <CalibrationOffset>32768</CalibrationOffset>\n      <CalibrationSlope>-65.7</CalibrationSlope>\n      <ParameterType>7</ParameterType>\n      <Description>Collision Cell Lens 3</Description>\n      <Linked>Equation</Linked>\n      <Unlinked>Operator</Unlinked>\n      <Location>Compound</Location>\n    </ParaRow>\n    <ParaRow Row=\"21\">\n      <Parameter>CC L4</Parameter>\n      <Channal>16</Channal>\n      <UserMin>0</UserMin>\n      <UserMax>400</UserMax>\n      <UserDefault>62</UserDefault>\n      <CalibrationOffset>32768</CalibrationOffset>\n      <CalibrationSlope>-65.7</CalibrationSlope>\n      <ParameterType>7</ParameterType>\n      <Description>Collision Cell Lens 4</Description>\n      <Linked>Equation</Linked>\n      <Unlinked>Operator</Unlinked>\n      <Location>Compound</Location>\n    </ParaRow>\n    <ParaRow Row=\"22\">\n      <Parameter>Q2</Parameter>\n      <Channal>8</Channal>\n      <UserMin>0</UserMin>\n      <UserMax>150</UserMax>\n      <UserDefault>52</UserDefault>\n      <CalibrationOffset>32756</CalibrationOffset>\n      <CalibrationSlope>-131.3</CalibrationSlope>\n      <ParameterType>11</ParameterType>\n      <Description>Quadrupole 2</Description>\n      <Linked>Equation</Linked>\n      <Unlinked>Equation</Unlinked>\n      <Location>Resolution</Location>\n    </ParaRow>\n    <ParaRow Row=\"23\">\n      <Parameter>ID</Parameter>\n      <Channal>17</Channal>\n      <UserMin>0</UserMin>\n      <UserMax>400</UserMax>\n      <UserDefault>110</UserDefault>\n      <CalibrationOffset>32768</CalibrationOffset>\n      <CalibrationSlope>-65.8</CalibrationSlope>\n      <ParameterType>7</ParameterType>\n      <Description>Detector Deflector</Description>\n      <Linked>Equation</Linked>\n      <Unlinked>Equation</Unlinked>\n      <Location>Compound</Location>\n    </ParaRow>\n    <ParaRow Row=\"24\">\n      <Parameter>DISC</Parameter>\n      <Channal>32</Channal>\n      <UserMin>10</UserMin>\n      <UserMax>2000</UserMax>\n      <UserDefault>15</UserDefault>\n      <CalibrationOffset>-5</CalibrationOffset>\n      <CalibrationSlope>1.23</CalibrationSlope>\n      <ParameterType>18</ParameterType>\n      <Description>Discriminator</Description>\n      <Linked>Fixed</Linked>\n      <Unlinked>Fixed</Unlinked>\n      <Location>Detector</Location>\n    </ParaRow>\n    <ParaRow Row=\"25\">\n      <Parameter>DV</Parameter>\n      <Channal>34</Channal>\n      <UserMin>1600</UserMin>\n      <UserMax>3500</UserMax>\n      <UserDefault>2000</UserDefault>\n      <CalibrationOffset>0</CalibrationOffset>\n      <CalibrationSlope>0.415</CalibrationSlope>\n      <ParameterType>18</ParameterType>\n      <Description>Detector Voltage</Description>\n      <Linked>Operator</Linked>\n      <Unlinked>Operator</Unlinked>\n      <Location>Detector</Location>\n    </ParaRow>\n    <ParaRow Row=\"26\">\n      <Parameter>DET horn</Parameter>\n      <Channal>200</Channal>\n      <UserMin>0</UserMin>\n      <UserMax>5500</UserMax>\n      <UserDefault>5500</UserDefault>\n      <CalibrationOffset>0</CalibrationOffset>\n      <CalibrationSlope>0.415</CalibrationSlope>\n      <ParameterType>16</ParameterType>\n      <Description>Detector Horn</Description>\n      <Linked>Fixed</Linked>\n      <Unlinked>Fixed</Unlinked>\n      <Location>Detector</Location>\n    </ParaRow>\n    <ParaRow Row=\"27\">\n      <Parameter>LS400A</Parameter>\n      <Channal>36</Channal>\n      <UserMin>0</UserMin>\n      <UserMax>420</UserMax>\n      <UserDefault>420</UserDefault>\n      <CalibrationOffset>0</CalibrationOffset>\n      <CalibrationSlope>8.4</CalibrationSlope>\n      <ParameterType>64</ParameterType>\n      <Description>Lens Power Supply A +400</Description>\n      <Linked>\n      </Linked>\n      <Unlinked>\n      </Unlinked>\n      <Location>\n      </Location>\n    </ParaRow>\n    <ParaRow Row=\"28\">\n      <Parameter>LS-400A</Parameter>\n      <Channal>37</Channal>\n      <UserMin>-420</UserMin>\n      <UserMax>-55</UserMax>\n      <UserDefault>-420</UserDefault>\n      <CalibrationOffset>-433</CalibrationOffset>\n      <CalibrationSlope>-8.4</CalibrationSlope>\n      <ParameterType>64</ParameterType>\n      <Description>Lens Power Supply A -400</Description>\n      <Linked>\n      </Linked>\n      <Unlinked>\n      </Unlinked>\n      <Location>\n      </Location>\n    </ParaRow>\n    <ParaRow Row=\"29\">\n      <Parameter>LS400B</Parameter>\n      <Channal>38</Channal>\n      <UserMin>0</UserMin>\n      <UserMax>420</UserMax>\n      <UserDefault>420</UserDefault>\n      <CalibrationOffset>0</CalibrationOffset>\n      <CalibrationSlope>8.4</CalibrationSlope>\n      <ParameterType>64</ParameterType>\n      <Description>Lens Power Supply B +400</Description>\n      <Linked>\n      </Linked>\n      <Unlinked>\n      </Unlinked>\n      <Location>\n      </Location>\n    </ParaRow>\n    <ParaRow Row=\"30\">\n      <Parameter>LS-400B</Parameter>\n      <Channal>39</Channal>\n      <UserMin>-420</UserMin>\n      <UserMax>-55</UserMax>\n      <UserDefault>-420</UserDefault>\n      <CalibrationOffset>-433</CalibrationOffset>\n      <CalibrationSlope>-8.4</CalibrationSlope>\n      <ParameterType>64</ParameterType>\n      <Description>Lens Power Supply B  -400</Description>\n      <Linked>\n      </Linked>\n      <Unlinked>\n      </Unlinked>\n      <Location>\n      </Location>\n    </ParaRow>\n    <ParaRow Row=\"31\">\n      <Parameter>QPS800</Parameter>\n      <Channal>40</Channal>\n      <UserMin>110</UserMin>\n      <UserMax>600</UserMax>\n      <UserDefault>600</UserDefault>\n      <CalibrationOffset>0</CalibrationOffset>\n      <CalibrationSlope>4.25</CalibrationSlope>\n      <ParameterType>64</ParameterType>\n      <Description>Quad Power Supply +800</Description>\n      <Linked>\n      </Linked>\n      <Unlinked>\n      </Unlinked>\n      <Location>\n      </Location>\n    </ParaRow>\n    <ParaRow Row=\"32\">\n      <Parameter>QPS-800</Parameter>\n      <Channal>41</Channal>\n      <UserMin>-110</UserMin>\n      <UserMax>-110</UserMax>\n      <UserDefault>-600</UserDefault>\n      <CalibrationOffset>-433</CalibrationOffset>\n      <CalibrationSlope>-4.2</CalibrationSlope>\n      <ParameterType>64</ParameterType>\n      <Description>Quad Power Supply -800</Description>\n      <Linked>\n      </Linked>\n      <Unlinked>\n      </Unlinked>\n      <Location>\n      </Location>\n    </ParaRow>\n    <ParaRow Row=\"33\">\n      <Parameter>DG</Parameter>\n      <Channal>26</Channal>\n      <UserMin>50</UserMin>\n      <UserMax>300</UserMax>\n      <UserDefault>80</UserDefault>\n      <CalibrationOffset>0</CalibrationOffset>\n      <CalibrationSlope>32.765</CalibrationSlope>\n      <ParameterType>32</ParameterType>\n      <Description>Drying Gas</Description>\n      <Linked>Operator</Linked>\n      <Unlinked>Operator</Unlinked>\n      <Location>Source</Location>\n    </ParaRow>\n    <ParaRow Row=\"34\">\n      <Parameter>NG1</Parameter>\n      <Channal>27</Channal>\n      <UserMin>0</UserMin>\n      <UserMax>450</UserMax>\n      <UserDefault>0</UserDefault>\n      <CalibrationOffset>0</CalibrationOffset>\n      <CalibrationSlope>32.765</CalibrationSlope>\n      <ParameterType>32</ParameterType>\n      <Description>Nebulizer Gas 1</Description>\n      <Linked>Operator</Linked>\n      <Unlinked>Operator</Unlinked>\n      <Location>Source</Location>\n    </ParaRow>\n    <ParaRow Row=\"35\">\n      <Parameter>HG1</Parameter>\n      <Channal>29</Channal>\n      <UserMin>0</UserMin>\n      <UserMax>350</UserMax>\n      <UserDefault>0</UserDefault>\n      <CalibrationOffset>0</CalibrationOffset>\n      <CalibrationSlope>32.765</CalibrationSlope>\n      <ParameterType>32</ParameterType>\n      <Description>Heating Gas 1</Description>\n      <Linked>Equation</Linked>\n      <Unlinked>Equation</Unlinked>\n      <Location>Source</Location>\n    </ParaRow>\n    <ParaRow Row=\"36\">\n      <Parameter>NG2</Parameter>\n      <Channal>28</Channal>\n      <UserMin>0</UserMin>\n      <UserMax>450</UserMax>\n      <UserDefault>0</UserDefault>\n      <CalibrationOffset>0</CalibrationOffset>\n      <CalibrationSlope>32.765</CalibrationSlope>\n      <ParameterType>32</ParameterType>\n      <Description>Nebulizer Gas 2</Description>\n      <Linked>Operator</Linked>\n      <Unlinked>Operator</Unlinked>\n      <Location>Source</Location>\n    </ParaRow>\n    <ParaRow Row=\"37\">\n      <Parameter>HG2</Parameter>\n      <Channal>30</Channal>\n      <UserMin>0</UserMin>\n      <UserMax>350</UserMax>\n      <UserDefault>0</UserDefault>\n      <CalibrationOffset>0</CalibrationOffset>\n      <CalibrationSlope>32.765</CalibrationSlope>\n      <ParameterType>32</ParameterType>\n      <Description>Heating Gas 2</Description>\n      <Linked>Equation</Linked>\n      <Unlinked>Equation</Unlinked>\n      <Location>Source</Location>\n    </ParaRow>\n    <ParaRow Row=\"38\">\n      <Parameter>CC P</Parameter>\n      <Channal>43</Channal>\n      <UserMin>0</UserMin>\n      <UserMax>500</UserMax>\n      <UserDefault>0</UserDefault>\n      <CalibrationOffset>0</CalibrationOffset>\n      <CalibrationSlope>32.765</CalibrationSlope>\n      <ParameterType>6</ParameterType>\n      <Description>Collision Pressure</Description>\n      <Linked>Fixed</Linked>\n      <Unlinked>Fixed</Unlinked>\n      <Location>Compound</Location>\n    </ParaRow>\n    <ParaRow Row=\"39\">\n      <Parameter>SX</Parameter>\n      <Channal>42</Channal>\n      <UserMin>0</UserMin>\n      <UserMax>500</UserMax>\n      <UserDefault>500</UserDefault>\n      <CalibrationOffset>0</CalibrationOffset>\n      <CalibrationSlope>32.765</CalibrationSlope>\n      <ParameterType>32</ParameterType>\n      <Description>Source Exhaust</Description>\n      <Linked>Fixed</Linked>\n      <Unlinked>Fixed</Unlinked>\n      <Location>Source</Location>\n    </ParaRow>\n    <ParaRow Row=\"40\">\n      <Parameter>ISV2</Parameter>\n      <Channal>204</Channal>\n      <UserMin>-5850</UserMin>\n      <UserMax>0</UserMax>\n      <UserDefault>0</UserDefault>\n      <CalibrationOffset>0</CalibrationOffset>\n      <CalibrationSlope>0.0436</CalibrationSlope>\n      <ParameterType>34</ParameterType>\n      <Description>ElectroSpray V2</Description>\n      <Linked>Operator</Linked>\n      <Unlinked>Operator</Unlinked>\n      <Location>Source</Location>\n    </ParaRow>\n    <ParaRow Row=\"41\">\n      <Parameter>ISV1</Parameter>\n      <Channal>203</Channal>\n      <UserMin>-5850</UserMin>\n      <UserMax>0</UserMax>\n      <UserDefault>0</UserDefault>\n      <CalibrationOffset>0</CalibrationOffset>\n      <CalibrationSlope>0.0436</CalibrationSlope>\n      <ParameterType>34</ParameterType>\n      <Description>ElectroSpray V1</Description>\n      <Linked>Operator</Linked>\n      <Unlinked>Operator</Unlinked>\n      <Location>Source</Location>\n    </ParaRow>\n    <ParaRow Row=\"42\">\n      <Parameter>CD</Parameter>\n      <Channal>202</Channal>\n      <UserMin>-5</UserMin>\n      <UserMax>0</UserMax>\n      <UserDefault>0</UserDefault>\n      <CalibrationOffset>0</CalibrationOffset>\n      <CalibrationSlope>51</CalibrationSlope>\n      <ParameterType>34</ParameterType>\n      <Description>Corona Discharge</Description>\n      <Linked>Operator</Linked>\n      <Unlinked>Operator</Unlinked>\n      <Location>Source</Location>\n    </ParaRow>\n    <ParaRow Row=\"43\">\n      <Parameter>CAP</Parameter>\n      <Channal>201</Channal>\n      <UserMin>-1100</UserMin>\n      <UserMax>0</UserMax>\n      <UserDefault>-1000</UserDefault>\n      <CalibrationOffset>0</CalibrationOffset>\n      <CalibrationSlope>0.22</CalibrationSlope>\n      <ParameterType>34</ParameterType>\n      <Description>Curtain Cap</Description>\n      <Linked>Fixed</Linked>\n      <Unlinked>Fixed</Unlinked>\n      <Location>Source</Location>\n    </ParaRow>\n    <ParaRow Row=\"44\">\n      <Parameter>HSID T</Parameter>\n      <Channal>81</Channal>\n      <UserMin>0</UserMin>\n      <UserMax>320</UserMax>\n      <UserDefault>200</UserDefault>\n      <CalibrationOffset>0</CalibrationOffset>\n      <CalibrationSlope>1</CalibrationSlope>\n      <ParameterType>32</ParameterType>\n      <Description>HSID Temperature</Description>\n      <Linked>Operator</Linked>\n      <Unlinked>Operator</Unlinked>\n      <Location>Source</Location>\n    </ParaRow>\n    <ParaRow Row=\"45\">\n      <Parameter>P1 T</Parameter>\n      <Channal>86</Channal>\n      <UserMin>0</UserMin>\n      <UserMax>500</UserMax>\n      <UserDefault>0</UserDefault>\n      <CalibrationOffset>0</CalibrationOffset>\n      <CalibrationSlope>1</CalibrationSlope>\n      <ParameterType>32</ParameterType>\n      <Description>Source 1 Temp</Description>\n      <Linked>Operator</Linked>\n      <Unlinked>Operator</Unlinked>\n      <Location>Source</Location>\n    </ParaRow>\n    <ParaRow Row=\"46\">\n      <Parameter>P2 T</Parameter>\n      <Channal>84</Channal>\n      <UserMin>0</UserMin>\n      <UserMax>500</UserMax>\n      <UserDefault>0</UserDefault>\n      <CalibrationOffset>0</CalibrationOffset>\n      <CalibrationSlope>1</CalibrationSlope>\n      <ParameterType>32</ParameterType>\n      <Description>Source 2 Temp</Description>\n      <Linked>Operator</Linked>\n      <Unlinked>Operator</Unlinked>\n      <Location>Source</Location>\n    </ParaRow>\n  </ScanType>", "<ScanType name=\"Q2Positive\">\n    <ParaRow Row=\"1\">\n      <Parameter>Q1 RF</Parameter>\n      <Channal>1</Channal>\n      <UserMin>10</UserMin>\n      <UserMax>2150</UserMax>\n      <UserDefault>400</UserDefault>\n      <CalibrationOffset>0</CalibrationOffset>\n      <CalibrationSlope>218.45</CalibrationSlope>\n      <ParameterType>64</ParameterType>\n      <Description>Quadrupole 1 RF</Description>\n      <Linked>\n      </Linked>\n      <Unlinked>\n      </Unlinked>\n      <Location>\n      </Location>\n    </ParaRow>\n    <ParaRow Row=\"2\">\n      <Parameter>Q1 DC</Parameter>\n      <Channal>4</Channal>\n      <UserMin>10</UserMin>\n      <UserMax>2150</UserMax>\n      <UserDefault>600</UserDefault>\n      <CalibrationOffset>0</CalibrationOffset>\n      <CalibrationSlope>218.45</CalibrationSlope>\n      <ParameterType>64</ParameterType>\n      <Description>Quadrupole 1 DC</Description>\n      <Linked>\n      </Linked>\n      <Unlinked>\n      </Unlinked>\n      <Location>\n      </Location>\n    </ParaRow>\n    <ParaRow Row=\"3\">\n      <Parameter>Q1 RR</Parameter>\n      <Channal>7</Channal>\n      <UserMin>0</UserMin>\n      <UserMax>64000</UserMax>\n      <UserDefault>32768</UserDefault>\n      <CalibrationOffset>32768</CalibrationOffset>\n      <CalibrationSlope>1</CalibrationSlope>\n      <ParameterType>64</ParameterType>\n      <Description>Quadrupole 1 PW</Description>\n      <Linked>\n      </Linked>\n      <Unlinked>\n      </Unlinked>\n      <Location>\n      </Location>\n    </ParaRow>\n    <ParaRow Row=\"4\">\n      <Parameter>Q2 RF</Parameter>\n      <Channal>2</Channal>\n      <UserMin>10</UserMin>\n      <UserMax>2150</UserMax>\n      <UserDefault>400</UserDefault>\n      <CalibrationOffset>0</CalibrationOffset>\n      <CalibrationSlope>218.45</CalibrationSlope>\n      <ParameterType>64</ParameterType>\n      <Description>Quadrupole 2 RF</Description>\n      <Linked>\n      </Linked>\n      <Unlinked>\n      </Unlinked>\n      <Location>\n      </Location>\n    </ParaRow>\n    <ParaRow Row=\"5\">\n      <Parameter>Q2 DC</Parameter>\n      <Channal>5</Channal>\n      <UserMin>10</UserMin>\n      <UserMax>2150</UserMax>\n      <UserDefault>600</UserDefault>\n      <CalibrationOffset>0</CalibrationOffset>\n      <CalibrationSlope>218.45</CalibrationSlope>\n      <ParameterType>64</ParameterType>\n      <Description>Quadrupole 2 DC</Description>\n      <Linked>\n      </Linked>\n      <Unlinked>\n      </Unlinked>\n      <Location>\n      </Location>\n    </ParaRow>\n    <ParaRow Row=\"6\">\n      <Parameter>Q2 RR</Parameter>\n      <Channal>9</Channal>\n      <UserMin>0</UserMin>\n      <UserMax>64000</UserMax>\n      <UserDefault>32768</UserDefault>\n      <CalibrationOffset>32768</CalibrationOffset>\n      <CalibrationSlope>1</CalibrationSlope>\n      <ParameterType>64</ParameterType>\n      <Description>Quadrupole 2 PW</Description>\n      <Linked>\n      </Linked>\n      <Unlinked>\n      </Unlinked>\n      <Location>\n      </Location>\n    </ParaRow>\n    <ParaRow Row=\"7\">\n      <Parameter>M1 RF</Parameter>\n      <Channal>3</Channal>\n      <UserMin>0</UserMin>\n      <UserMax>600</UserMax>\n      <UserDefault>500</UserDefault>\n      <CalibrationOffset>0</CalibrationOffset>\n      <CalibrationSlope>14.7</CalibrationSlope>\n      <ParameterType>6</ParameterType>\n      <Description>Multipole 1 RF</Description>\n      <Linked>Fixed</Linked>\n      <Unlinked>Operator</Unlinked>\n      <Location>Compound</Location>\n    </ParaRow>\n    <ParaRow Row=\"8\">\n      <Parameter>EV</Parameter>\n      <Channal>20</Channal>\n      <UserMin>0</UserMin>\n      <UserMax>200</UserMax>\n      <UserDefault>100</UserDefault>\n      <CalibrationOffset>32768</CalibrationOffset>\n      <CalibrationSlope>-65.7</CalibrationSlope>\n      <ParameterType>7</ParameterType>\n      <Description>Entrance Voltage</Description>\n      <Linked>Operator</Linked>\n      <Unlinked>Operator</Unlinked>\n      <Location>Compound</Location>\n    </ParaRow>\n    <ParaRow Row=\"9\">\n      <Parameter>ED</Parameter>\n      <Channal>21</Channal>\n      <UserMin>0</UserMin>\n      <UserMax>200</UserMax>\n      <UserDefault>90</UserDefault>\n      <CalibrationOffset>32768</CalibrationOffset>\n      <CalibrationSlope>-65.5</CalibrationSlope>\n      <ParameterType>7</ParameterType>\n      <Description>Entrance Deflector</Description>\n      <Linked>Operator</Linked>\n      <Unlinked>Operator</Unlinked>\n      <Location>Compound</Location>\n    </ParaRow>\n    <ParaRow Row=\"10\">\n      <Parameter>M1</Parameter>\n      <Channal>19</Channal>\n      <UserMin>-10</UserMin>\n      <UserMax>5</UserMax>\n      <UserDefault>-1</UserDefault>\n      <CalibrationOffset>32768</CalibrationOffset>\n      <CalibrationSlope>-65.6</CalibrationSlope>\n      <ParameterType>7</ParameterType>\n      <Description>Multipole 1</Description>\n      <Linked>Equation</Linked>\n      <Unlinked>Equation</Unlinked>\n      <Location>Compound</Location>\n    </ParaRow>\n    <ParaRow Row=\"11\">\n      <Parameter>L1</Parameter>\n      <Channal>18</Channal>\n      <UserMin>-10</UserMin>\n      <UserMax>5</UserMax>\n      <UserDefault>-2</UserDefault>\n      <CalibrationOffset>32760</CalibrationOffset>\n      <CalibrationSlope>-65.9</CalibrationSlope>\n      <ParameterType>7</ParameterType>\n      <Description>Multipole Lens 1</Description>\n      <Linked>Equation</Linked>\n      <Unlinked>Equation</Unlinked>\n      <Location>Compound</Location>\n    </ParaRow>\n    <ParaRow Row=\"12\">\n      <Parameter>M2</Parameter>\n      <Channal>22</Channal>\n      <UserMin>-10</UserMin>\n      <UserMax>5</UserMax>\n      <UserDefault>-3</UserDefault>\n      <CalibrationOffset>32768</CalibrationOffset>\n      <CalibrationSlope>-66</CalibrationSlope>\n      <ParameterType>7</ParameterType>\n      <Description>Multipole 2</Description>\n      <Linked>Fixed</Linked>\n      <Unlinked>Fixed</Unlinked>\n      <Location>Compound</Location>\n    </ParaRow>\n    <ParaRow Row=\"13\">\n      <Parameter>L2</Parameter>\n      <Channal>11</Channal>\n      <UserMin>-10</UserMin>\n      <UserMax>5</UserMax>\n      <UserDefault>-4</UserDefault>\n      <CalibrationOffset>32768</CalibrationOffset>\n      <CalibrationSlope>-65.9</CalibrationSlope>\n      <ParameterType>7</ParameterType>\n      <Description>Multipole Lens 2</Description>\n      <Linked>Equation</Linked>\n      <Unlinked>Equation</Unlinked>\n      <Location>Compound</Location>\n    </ParaRow>\n    <ParaRow Row=\"14\">\n      <Parameter>PF</Parameter>\n      <Channal>12</Channal>\n      <UserMin>-50</UserMin>\n      <UserMax>5</UserMax>\n      <UserDefault>-15</UserDefault>\n      <CalibrationOffset>32768</CalibrationOffset>\n      <CalibrationSlope>-65.8</CalibrationSlope>\n      <ParameterType>7</ParameterType>\n      <Description>Prefilter 1</Description>\n      <Linked>Equation</Linked>\n      <Unlinked>Operator</Unlinked>\n      <Location>Compound</Location>\n    </ParaRow>\n    <ParaRow Row=\"15\">\n      <Parameter>Q1</Parameter>\n      <Channal>6</Channal>\n      <UserMin>-10</UserMin>\n      <UserMax>0</UserMax>\n      <UserDefault>-4.5</UserDefault>\n      <CalibrationOffset>32755</CalibrationOffset>\n      <CalibrationSlope>-131.3</CalibrationSlope>\n      <ParameterType>11</ParameterType>\n      <Description>Quadrupole 1</Description>\n      <Linked>Equation</Linked>\n      <Unlinked>Operator</Unlinked>\n      <Location>Resolution</Location>\n    </ParaRow>\n    <ParaRow Row=\"16\">\n      <Parameter>CC L1</Parameter>\n      <Channal>13</Channal>\n      <UserMin>-100</UserMin>\n      <UserMax>10</UserMax>\n      <UserDefault>-10</UserDefault>\n      <CalibrationOffset>32768</CalibrationOffset>\n      <CalibrationSlope>-65.8</CalibrationSlope>\n      <ParameterType>7</ParameterType>\n      <Description>Collision Cell Lens 1</Description>\n      <Linked>Equation</Linked>\n      <Unlinked>Operator</Unlinked>\n      <Location>Compound</Location>\n    </ParaRow>\n    <ParaRow Row=\"17\">\n      <Parameter>CC L2</Parameter>\n      <Channal>14</Channal>\n      <UserMin>-400</UserMin>\n      <UserMax>-10</UserMax>\n      <UserDefault>-100</UserDefault>\n      <CalibrationOffset>32768</CalibrationOffset>\n      <CalibrationSlope>-65.8</CalibrationSlope>\n      <ParameterType>7</ParameterType>\n      <Description>Collision Cell Lens 2</Description>\n      <Linked>Operator</Linked>\n      <Unlinked>Operator</Unlinked>\n      <Location>Compound</Location>\n    </ParaRow>\n    <ParaRow Row=\"18\">\n      <Parameter>CC</Parameter>\n      <Channal>23</Channal>\n      <UserMin>-150</UserMin>\n      <UserMax>0</UserMax>\n      <UserDefault>-15</UserDefault>\n      <CalibrationOffset>32768</CalibrationOffset>\n      <CalibrationSlope>-65.8</CalibrationSlope>\n      <ParameterType>7</ParameterType>\n      <Description>Collision Energy</Description>\n      <Linked>Fixed</Linked>\n      <Unlinked>Operator</Unlinked>\n      <Location>Compound</Location>\n    </ParaRow>\n    <ParaRow Row=\"19\">\n      <Parameter>CC AF</Parameter>\n      <Channal>10</Channal>\n      <UserMin>0</UserMin>\n      <UserMax>400</UserMax>\n      <UserDefault>100</UserDefault>\n      <CalibrationOffset>32768</CalibrationOffset>\n      <CalibrationSlope>-65.8</CalibrationSlope>\n      <ParameterType>7</ParameterType>\n      <Description>Axial Field</Description>\n      <Linked>Fixed</Linked>\n      <Unlinked>Fixed</Unlinked>\n      <Location>Compound</Location>\n    </ParaRow>\n    <ParaRow Row=\"20\">\n      <Parameter>CC L3</Parameter>\n      <Channal>15</Channal>\n      <UserMin>-160</UserMin>\n      <UserMax>0</UserMax>\n      <UserDefault>-16</UserDefault>\n      <CalibrationOffset>32768</CalibrationOffset>\n      <CalibrationSlope>-65.7</CalibrationSlope>\n      <ParameterType>7</ParameterType>\n      <Description>Collision Cell Lens 3</Description>\n      <Linked>Equation</Linked>\n      <Unlinked>Equation</Unlinked>\n      <Location>Compound</Location>\n    </ParaRow>\n    <ParaRow Row=\"21\">\n      <Parameter>CC L4</Parameter>\n      <Channal>16</Channal>\n      <UserMin>-400</UserMin>\n      <UserMax>0</UserMax>\n      <UserDefault>-27</UserDefault>\n      <CalibrationOffset>32768</CalibrationOffset>\n      <CalibrationSlope>-65.7</CalibrationSlope>\n      <ParameterType>7</ParameterType>\n      <Description>Collision Cell Lens 4</Description>\n      <Linked>Equation</Linked>\n      <Unlinked>Operator</Unlinked>\n      <Location>Compound</Location>\n    </ParaRow>\n    <ParaRow Row=\"22\">\n      <Parameter>Q2</Parameter>\n      <Channal>8</Channal>\n      <UserMin>-150</UserMin>\n      <UserMax>0</UserMax>\n      <UserDefault>-17</UserDefault>\n      <CalibrationOffset>32756</CalibrationOffset>\n      <CalibrationSlope>-131.3</CalibrationSlope>\n      <ParameterType>11</ParameterType>\n      <Description>Quadrupole 2</Description>\n      <Linked>Equation</Linked>\n      <Unlinked>Equation</Unlinked>\n      <Location>Resolution</Location>\n    </ParaRow>\n    <ParaRow Row=\"23\">\n      <Parameter>ID</Parameter>\n      <Channal>17</Channal>\n      <UserMin>-400</UserMin>\n      <UserMax>0</UserMax>\n      <UserDefault>-105</UserDefault>\n      <CalibrationOffset>32768</CalibrationOffset>\n      <CalibrationSlope>-65.8</CalibrationSlope>\n      <ParameterType>7</ParameterType>\n      <Description>Detector Deflector</Description>\n      <Linked>Equation</Linked>\n      <Unlinked>Equation</Unlinked>\n      <Location>Compound</Location>\n    </ParaRow>\n    <ParaRow Row=\"24\">\n      <Parameter>DISC</Parameter>\n      <Channal>32</Channal>\n      <UserMin>10</UserMin>\n      <UserMax>2000</UserMax>\n      <UserDefault>15</UserDefault>\n      <CalibrationOffset>-5</CalibrationOffset>\n      <CalibrationSlope>1.23</CalibrationSlope>\n      <ParameterType>18</ParameterType>\n      <Description>Discriminator</Description>\n      <Linked>Fixed</Linked>\n      <Unlinked>Fixed</Unlinked>\n      <Location>Detector</Location>\n    </ParaRow>\n    <ParaRow Row=\"25\">\n      <Parameter>DV</Parameter>\n      <Channal>34</Channal>\n      <UserMin>1600</UserMin>\n      <UserMax>3500</UserMax>\n      <UserDefault>2000</UserDefault>\n      <CalibrationOffset>0</CalibrationOffset>\n      <CalibrationSlope>0.415</CalibrationSlope>\n      <ParameterType>18</ParameterType>\n      <Description>Detector Voltage</Description>\n      <Linked>Operator</Linked>\n      <Unlinked>Operator</Unlinked>\n      <Location>Detector</Location>\n    </ParaRow>\n    <ParaRow Row=\"26\">\n      <Parameter>DET horn</Parameter>\n      <Channal>200</Channal>\n      <UserMin>0</UserMin>\n      <UserMax>5500</UserMax>\n      <UserDefault>5500</UserDefault>\n      <CalibrationOffset>0</CalibrationOffset>\n      <CalibrationSlope>0.415</CalibrationSlope>\n      <ParameterType>16</ParameterType>\n      <Description>Detector Horn</Description>\n      <Linked>Fixed</Linked>\n      <Unlinked>Fixed</Unlinked>\n      <Location>Detector</Location>\n    </ParaRow>\n    <ParaRow Row=\"27\">\n      <Parameter>LS400A</Parameter>\n      <Channal>36</Channal>\n      <UserMin>0</UserMin>\n      <UserMax>420</UserMax>\n      <UserDefault>420</UserDefault>\n      <CalibrationOffset>0</CalibrationOffset>\n      <CalibrationSlope>8.4</CalibrationSlope>\n      <ParameterType>64</ParameterType>\n      <Description>Lens Power Supply A +400</Description>\n      <Linked>\n      </Linked>\n      <Unlinked>\n      </Unlinked>\n      <Location>\n      </Location>\n    </ParaRow>\n    <ParaRow Row=\"28\">\n      <Parameter>LS-400A</Parameter>\n      <Channal>37</Channal>\n      <UserMin>-420</UserMin>\n      <UserMax>-55</UserMax>\n      <UserDefault>-420</UserDefault>\n      <CalibrationOffset>-433</CalibrationOffset>\n      <CalibrationSlope>-8.4</CalibrationSlope>\n      <ParameterType>64</ParameterType>\n      <Description>Lens Power Supply A -400</Description>\n      <Linked>\n      </Linked>\n      <Unlinked>\n      </Unlinked>\n      <Location>\n      </Location>\n    </ParaRow>\n    <ParaRow Row=\"29\">\n      <Parameter>LS400B</Parameter>\n      <Channal>38</Channal>\n      <UserMin>0</UserMin>\n      <UserMax>420</UserMax>\n      <UserDefault>420</UserDefault>\n      <CalibrationOffset>0</CalibrationOffset>\n      <CalibrationSlope>8.4</CalibrationSlope>\n      <ParameterType>64</ParameterType>\n      <Description>Lens Power Supply B +400</Description>\n      <Linked>\n      </Linked>\n      <Unlinked>\n      </Unlinked>\n      <Location>\n      </Location>\n    </ParaRow>\n    <ParaRow Row=\"30\">\n      <Parameter>LS-400B</Parameter>\n      <Channal>39</Channal>\n      <UserMin>-420</UserMin>\n      <UserMax>-55</UserMax>\n      <UserDefault>-420</UserDefault>\n      <CalibrationOffset>-433</CalibrationOffset>\n      <CalibrationSlope>-8.4</CalibrationSlope>\n      <ParameterType>64</ParameterType>\n      <Description>Lens Power Supply B  -400</Description>\n      <Linked>\n      </Linked>\n      <Unlinked>\n      </Unlinked>\n      <Location>\n      </Location>\n    </ParaRow>\n    <ParaRow Row=\"31\">\n      <Parameter>QPS800</Parameter>\n      <Channal>40</Channal>\n      <UserMin>110</UserMin>\n      <UserMax>600</UserMax>\n      <UserDefault>600</UserDefault>\n      <CalibrationOffset>0</CalibrationOffset>\n      <CalibrationSlope>4.25</CalibrationSlope>\n      <ParameterType>64</ParameterType>\n      <Description>Quad Power Supply +800</Description>\n      <Linked>\n      </Linked>\n      <Unlinked>\n      </Unlinked>\n      <Location>\n      </Location>\n    </ParaRow>\n    <ParaRow Row=\"32\">\n      <Parameter>QPS-800</Parameter>\n      <Channal>41</Channal>\n      <UserMin>-110</UserMin>\n      <UserMax>-110</UserMax>\n      <UserDefault>-600</UserDefault>\n      <CalibrationOffset>-433</CalibrationOffset>\n      <CalibrationSlope>-4.2</CalibrationSlope>\n      <ParameterType>64</ParameterType>\n      <Description>Quad Power Supply -800</Description>\n      <Linked>\n      </Linked>\n      <Unlinked>\n      </Unlinked>\n      <Location>\n      </Location>\n    </ParaRow>\n    <ParaRow Row=\"33\">\n      <Parameter>DG</Parameter>\n      <Channal>26</Channal>\n      <UserMin>50</UserMin>\n      <UserMax>300</UserMax>\n      <UserDefault>80</UserDefault>\n      <CalibrationOffset>0</CalibrationOffset>\n      <CalibrationSlope>32.765</CalibrationSlope>\n      <ParameterType>32</ParameterType>\n      <Description>Drying Gas</Description>\n      <Linked>Operator</Linked>\n      <Unlinked>Operator</Unlinked>\n      <Location>Source</Location>\n    </ParaRow>\n    <ParaRow Row=\"34\">\n      <Parameter>NG1</Parameter>\n      <Channal>27</Channal>\n      <UserMin>0</UserMin>\n      <UserMax>450</UserMax>\n      <UserDefault>0</UserDefault>\n      <CalibrationOffset>0</CalibrationOffset>\n      <CalibrationSlope>32.765</CalibrationSlope>\n      <ParameterType>32</ParameterType>\n      <Description>Nebulizer Gas 1</Description>\n      <Linked>Operator</Linked>\n      <Unlinked>Operator</Unlinked>\n      <Location>Source</Location>\n    </ParaRow>\n    <ParaRow Row=\"35\">\n      <Parameter>HG1</Parameter>\n      <Channal>29</Channal>\n      <UserMin>0</UserMin>\n      <UserMax>350</UserMax>\n      <UserDefault>0</UserDefault>\n      <CalibrationOffset>0</CalibrationOffset>\n      <CalibrationSlope>32.765</CalibrationSlope>\n      <ParameterType>32</ParameterType>\n      <Description>Heating Gas 1</Description>\n      <Linked>Equation</Linked>\n      <Unlinked>Equation</Unlinked>\n      <Location>Source</Location>\n    </ParaRow>\n    <ParaRow Row=\"36\">\n      <Parameter>NG2</Parameter>\n      <Channal>28</Channal>\n      <UserMin>0</UserMin>\n      <UserMax>450</UserMax>\n      <UserDefault>0</UserDefault>\n      <CalibrationOffset>0</CalibrationOffset>\n      <CalibrationSlope>32.765</CalibrationSlope>\n      <ParameterType>32</ParameterType>\n      <Description>Nebulizer Gas 2</Description>\n      <Linked>Operator</Linked>\n      <Unlinked>Operator</Unlinked>\n      <Location>Source</Location>\n    </ParaRow>\n    <ParaRow Row=\"37\">\n      <Parameter>HG2</Parameter>\n      <Channal>30</Channal>\n      <UserMin>0</UserMin>\n      <UserMax>350</UserMax>\n      <UserDefault>0</UserDefault>\n      <CalibrationOffset>0</CalibrationOffset>\n      <CalibrationSlope>32.765</CalibrationSlope>\n      <ParameterType>32</ParameterType>\n      <Description>Heating Gas 2</Description>\n      <Linked>Equation</Linked>\n      <Unlinked>Equation</Unlinked>\n      <Location>Source</Location>\n    </ParaRow>\n    <ParaRow Row=\"38\">\n      <Parameter>CC P</Parameter>\n      <Channal>43</Channal>\n      <UserMin>0</UserMin>\n      <UserMax>500</UserMax>\n      <UserDefault>410</UserDefault>\n      <CalibrationOffset>0</CalibrationOffset>\n      <CalibrationSlope>32.765</CalibrationSlope>\n      <ParameterType>6</ParameterType>\n      <Description>Collision Pressure</Description>\n      <Linked>Fixed</Linked>\n      <Unlinked>Operator</Unlinked>\n      <Location>Compound</Location>\n    </ParaRow>\n    <ParaRow Row=\"39\">\n      <Parameter>SX</Parameter>\n      <Channal>42</Channal>\n      <UserMin>0</UserMin>\n      <UserMax>500</UserMax>\n      <UserDefault>500</UserDefault>\n      <CalibrationOffset>0</CalibrationOffset>\n      <CalibrationSlope>32.765</CalibrationSlope>\n      <ParameterType>32</ParameterType>\n      <Description>Source Exhaust</Description>\n      <Linked>Fixed</Linked>\n      <Unlinked>Fixed</Unlinked>\n      <Location>Source</Location>\n    </ParaRow>\n    <ParaRow Row=\"40\">\n      <Parameter>ISV2</Parameter>\n      <Channal>204</Channal>\n      <UserMin>0</UserMin>\n      <UserMax>5850</UserMax>\n      <UserDefault>0</UserDefault>\n      <CalibrationOffset>0</CalibrationOffset>\n      <CalibrationSlope>0.0436</CalibrationSlope>\n      <ParameterType>34</ParameterType>\n      <Description>ElectroSpray V2</Description>\n      <Linked>Operator</Linked>\n      <Unlinked>Operator</Unlinked>\n      <Location>Source</Location>\n    </ParaRow>\n    <ParaRow Row=\"41\">\n      <Parameter>ISV1</Parameter>\n      <Channal>203</Channal>\n      <UserMin>0</UserMin>\n      <UserMax>5850</UserMax>\n      <UserDefault>0</UserDefault>\n      <CalibrationOffset>0</CalibrationOffset>\n      <CalibrationSlope>0.0436</CalibrationSlope>\n      <ParameterType>34</ParameterType>\n      <Description>ElectroSpray V1</Description>\n      <Linked>Operator</Linked>\n      <Unlinked>Operator</Unlinked>\n      <Location>Source</Location>\n    </ParaRow>\n    <ParaRow Row=\"42\">\n      <Parameter>CD</Parameter>\n      <Channal>202</Channal>\n      <UserMin>0</UserMin>\n      <UserMax>5</UserMax>\n      <UserDefault>0</UserDefault>\n      <CalibrationOffset>0</CalibrationOffset>\n      <CalibrationSlope>51</CalibrationSlope>\n      <ParameterType>34</ParameterType>\n      <Description>Corona Discharge</Description>\n      <Linked>Operator</Linked>\n      <Unlinked>Operator</Unlinked>\n      <Location>Source</Location>\n    </ParaRow>\n    <ParaRow Row=\"43\">\n      <Parameter>CAP</Parameter>\n      <Channal>201</Channal>\n      <UserMin>0</UserMin>\n      <UserMax>1100</UserMax>\n      <UserDefault>1000</UserDefault>\n      <CalibrationOffset>0</CalibrationOffset>\n      <CalibrationSlope>0.22</CalibrationSlope>\n      <ParameterType>34</ParameterType>\n      <Description>Curtain Cap</Description>\n      <Linked>Fixed</Linked>\n      <Unlinked>Fixed</Unlinked>\n      <Location>Source</Location>\n    </ParaRow>\n    <ParaRow Row=\"44\">\n      <Parameter>HSID T</Parameter>\n      <Channal>81</Channal>\n      <UserMin>0</UserMin>\n      <UserMax>320</UserMax>\n      <UserDefault>200</UserDefault>\n      <CalibrationOffset>0</CalibrationOffset>\n      <CalibrationSlope>1</CalibrationSlope>\n      <ParameterType>32</ParameterType>\n      <Description>HSID Temperature</Description>\n      <Linked>Operator</Linked>\n      <Unlinked>Operator</Unlinked>\n      <Location>Source</Location>\n    </ParaRow>\n    <ParaRow Row=\"45\">\n      <Parameter>P1 T</Parameter>\n      <Channal>86</Channal>\n      <UserMin>0</UserMin>\n      <UserMax>500</UserMax>\n      <UserDefault>0</UserDefault>\n      <CalibrationOffset>0</CalibrationOffset>\n      <CalibrationSlope>1</CalibrationSlope>\n      <ParameterType>32</ParameterType>\n      <Description>Source 1 Temp</Description>\n      <Linked>Operator</Linked>\n      <Unlinked>Operator</Unlinked>\n      <Location>Source</Location>\n    </ParaRow>\n    <ParaRow Row=\"46\">\n      <Parameter>P2 T</Parameter>\n      <Channal>84</Channal>\n      <UserMin>0</UserMin>\n      <UserMax>500</UserMax>\n      <UserDefault>0</UserDefault>\n      <CalibrationOffset>0</CalibrationOffset>\n      <CalibrationSlope>1</CalibrationSlope>\n      <ParameterType>32</ParameterType>\n      <Description>Source 2 Temp</Description>\n      <Linked>Operator</Linked>\n      <Unlinked>Operator</Unlinked>\n      <Location>Source</Location>\n    </ParaRow>\n  </ScanType>", "<ScanType name=\"Q2Negative\">\n    <ParaRow Row=\"1\">\n      <Parameter>Q1 RF</Parameter>\n      <Channal>1</Channal>\n      <UserMin>10</UserMin>\n      <UserMax>2150</UserMax>\n      <UserDefault>400</UserDefault>\n      <CalibrationOffset>0</CalibrationOffset>\n      <CalibrationSlope>218.45</CalibrationSlope>\n      <ParameterType>64</ParameterType>\n      <Description>Quadrupole 1 RF</Description>\n      <Linked>\n      </Linked>\n      <Unlinked>\n      </Unlinked>\n      <Location>\n      </Location>\n    </ParaRow>\n    <ParaRow Row=\"2\">\n      <Parameter>Q1 DC</Parameter>\n      <Channal>4</Channal>\n      <UserMin>10</UserMin>\n      <UserMax>2150</UserMax>\n      <UserDefault>600</UserDefault>\n      <CalibrationOffset>0</CalibrationOffset>\n      <CalibrationSlope>218.45</CalibrationSlope>\n      <ParameterType>64</ParameterType>\n      <Description>Quadrupole 1 DC</Description>\n      <Linked>\n      </Linked>\n      <Unlinked>\n      </Unlinked>\n      <Location>\n      </Location>\n    </ParaRow>\n    <ParaRow Row=\"3\">\n      <Parameter>Q1 RR</Parameter>\n      <Channal>7</Channal>\n      <UserMin>0</UserMin>\n      <UserMax>64000</UserMax>\n      <UserDefault>32768</UserDefault>\n      <CalibrationOffset>32768</CalibrationOffset>\n      <CalibrationSlope>1</CalibrationSlope>\n      <ParameterType>64</ParameterType>\n      <Description>Quadrupole 1 PW</Description>\n      <Linked>\n      </Linked>\n      <Unlinked>\n      </Unlinked>\n      <Location>\n      </Location>\n    </ParaRow>\n    <ParaRow Row=\"4\">\n      <Parameter>Q2 RF</Parameter>\n      <Channal>2</Channal>\n      <UserMin>10</UserMin>\n      <UserMax>2150</UserMax>\n      <UserDefault>400</UserDefault>\n      <CalibrationOffset>0</CalibrationOffset>\n      <CalibrationSlope>218.45</CalibrationSlope>\n      <ParameterType>64</ParameterType>\n      <Description>Quadrupole 2 RF</Description>\n      <Linked>\n      </Linked>\n      <Unlinked>\n      </Unlinked>\n      <Location>\n      </Location>\n    </ParaRow>\n    <ParaRow Row=\"5\">\n      <Parameter>Q2 DC</Parameter>\n      <Channal>5</Channal>\n      <UserMin>10</UserMin>\n      <UserMax>2150</UserMax>\n      <UserDefault>600</UserDefault>\n      <CalibrationOffset>0</CalibrationOffset>\n      <CalibrationSlope>218.45</CalibrationSlope>\n      <ParameterType>64</ParameterType>\n      <Description>Quadrupole 2 DC</Description>\n      <Linked>\n      </Linked>\n      <Unlinked>\n      </Unlinked>\n      <Location>\n      </Location>\n    </ParaRow>\n    <ParaRow Row=\"6\">\n      <Parameter>Q2 RR</Parameter>\n      <Channal>9</Channal>\n      <UserMin>0</UserMin>\n      <UserMax>64000</UserMax>\n      <UserDefault>32768</UserDefault>\n      <CalibrationOffset>32768</CalibrationOffset>\n      <CalibrationSlope>1</CalibrationSlope>\n      <ParameterType>64</ParameterType>\n      <Description>Quadrupole 2 PW</Description>\n      <Linked>\n      </Linked>\n      <Unlinked>\n      </Unlinked>\n      <Location>\n      </Location>\n    </ParaRow>\n    <ParaRow Row=\"7\">\n      <Parameter>M1 RF</Parameter>\n      <Channal>3</Channal>\n      <UserMin>0</UserMin>\n      <UserMax>600</UserMax>\n      <UserDefault>500</UserDefault>\n      <CalibrationOffset>0</CalibrationOffset>\n      <CalibrationSlope>14.7</CalibrationSlope>\n      <ParameterType>6</ParameterType>\n      <Description>Multipole 1 RF</Description>\n      <Linked>Fixed</Linked>\n      <Unlinked>Operator</Unlinked>\n      <Location>Compound</Location>\n    </ParaRow>\n    <ParaRow Row=\"8\">\n      <Parameter>EV</Parameter>\n      <Channal>20</Channal>\n      <UserMin>-200</UserMin>\n      <UserMax>0</UserMax>\n      <UserDefault>-100</UserDefault>\n      <CalibrationOffset>32768</CalibrationOffset>\n      <CalibrationSlope>-65.7</CalibrationSlope>\n      <ParameterType>7</ParameterType>\n      <Description>Entrance Voltage</Description>\n      <Linked>Operator</Linked>\n      <Unlinked>Operator</Unlinked>\n      <Location>Compound</Location>\n    </ParaRow>\n    <ParaRow Row=\"9\">\n      <Parameter>ED</Parameter>\n      <Channal>21</Channal>\n      <UserMin>-200</UserMin>\n      <UserMax>0</UserMax>\n      <UserDefault>-90</UserDefault>\n      <CalibrationOffset>32768</CalibrationOffset>\n      <CalibrationSlope>-65.5</CalibrationSlope>\n      <ParameterType>7</ParameterType>\n      <Description>Entrance Deflector</Description>\n      <Linked>Operator</Linked>\n      <Unlinked>Operator</Unlinked>\n      <Location>Compound</Location>\n    </ParaRow>\n    <ParaRow Row=\"10\">\n      <Parameter>M1</Parameter>\n      <Channal>19</Channal>\n      <UserMin>-5</UserMin>\n      <UserMax>10</UserMax>\n      <UserDefault>1</UserDefault>\n      <CalibrationOffset>32768</CalibrationOffset>\n      <CalibrationSlope>-65.6</CalibrationSlope>\n      <ParameterType>7</ParameterType>\n      <Description>Multipole 1</Description>\n      <Linked>Equation</Linked>\n      <Unlinked>Equation</Unlinked>\n      <Location>Compound</Location>\n    </ParaRow>\n    <ParaRow Row=\"11\">\n      <Parameter>L1</Parameter>\n      <Channal>18</Channal>\n      <UserMin>-5</UserMin>\n      <UserMax>10</UserMax>\n      <UserDefault>2</UserDefault>\n      <CalibrationOffset>32760</CalibrationOffset>\n      <CalibrationSlope>-65.9</CalibrationSlope>\n      <ParameterType>7</ParameterType>\n      <Description>Multipole Lens 1</Description>\n      <Linked>Equation</Linked>\n      <Unlinked>Equation</Unlinked>\n      <Location>Compound</Location>\n    </ParaRow>\n    <ParaRow Row=\"12\">\n      <Parameter>M2</Parameter>\n      <Channal>22</Channal>\n      <UserMin>-5</UserMin>\n      <UserMax>10</UserMax>\n      <UserDefault>3</UserDefault>\n      <CalibrationOffset>32768</CalibrationOffset>\n      <CalibrationSlope>-66</CalibrationSlope>\n      <ParameterType>7</ParameterType>\n      <Description>Multipole 2</Description>\n      <Linked>Fixed</Linked>\n      <Unlinked>Fixed</Unlinked>\n      <Location>Compound</Location>\n    </ParaRow>\n    <ParaRow Row=\"13\">\n      <Parameter>L2</Parameter>\n      <Channal>11</Channal>\n      <UserMin>-5</UserMin>\n      <UserMax>10</UserMax>\n      <UserDefault>4</UserDefault>\n      <CalibrationOffset>32768</CalibrationOffset>\n      <CalibrationSlope>-65.9</CalibrationSlope>\n      <ParameterType>7</ParameterType>\n      <Description>Multipole Lens 2</Description>\n      <Linked>Equation</Linked>\n      <Unlinked>Equation</Unlinked>\n      <Location>Compound</Location>\n    </ParaRow>\n    <ParaRow Row=\"14\">\n      <Parameter>PF</Parameter>\n      <Channal>12</Channal>\n      <UserMin>-5</UserMin>\n      <UserMax>50</UserMax>\n      <UserDefault>15</UserDefault>\n      <CalibrationOffset>32768</CalibrationOffset>\n      <CalibrationSlope>-65.8</CalibrationSlope>\n      <ParameterType>7</ParameterType>\n      <Description>Prefilter 1</Description>\n      <Linked>Equation</Linked>\n      <Unlinked>Operator</Unlinked>\n      <Location>Compound</Location>\n    </ParaRow>\n    <ParaRow Row=\"15\">\n      <Parameter>Q1</Parameter>\n      <Channal>6</Channal>\n      <UserMin>0</UserMin>\n      <UserMax>10</UserMax>\n      <UserDefault>4.5</UserDefault>\n      <CalibrationOffset>32755</CalibrationOffset>\n      <CalibrationSlope>-131.3</CalibrationSlope>\n      <ParameterType>11</ParameterType>\n      <Description>Quadrupole 1</Description>\n      <Linked>Equation</Linked>\n      <Unlinked>Operator</Unlinked>\n      <Location>Resolution</Location>\n    </ParaRow>\n    <ParaRow Row=\"16\">\n      <Parameter>CC L1</Parameter>\n      <Channal>13</Channal>\n      <UserMin>-10</UserMin>\n      <UserMax>100</UserMax>\n      <UserDefault>10</UserDefault>\n      <CalibrationOffset>32768</CalibrationOffset>\n      <CalibrationSlope>-65.8</CalibrationSlope>\n      <ParameterType>7</ParameterType>\n      <Description>Collision Cell Lens 1</Description>\n      <Linked>Equation</Linked>\n      <Unlinked>Operator</Unlinked>\n      <Location>Compound</Location>\n    </ParaRow>\n    <ParaRow Row=\"17\">\n      <Parameter>CC L2</Parameter>\n      <Channal>14</Channal>\n      <UserMin>0</UserMin>\n      <UserMax>400</UserMax>\n      <UserDefault>100</UserDefault>\n      <CalibrationOffset>32768</CalibrationOffset>\n      <CalibrationSlope>-65.8</CalibrationSlope>\n      <ParameterType>7</ParameterType>\n      <Description>Collision Cell Lens 2</Description>\n      <Linked>Operator</Linked>\n      <Unlinked>Operator</Unlinked>\n      <Location>Compound</Location>\n    </ParaRow>\n    <ParaRow Row=\"18\">\n      <Parameter>CC</Parameter>\n      <Channal>23</Channal>\n      <UserMin>0</UserMin>\n      <UserMax>150</UserMax>\n      <UserDefault>15</UserDefault>\n      <CalibrationOffset>32768</CalibrationOffset>\n      <CalibrationSlope>-65.8</CalibrationSlope>\n      <ParameterType>7</ParameterType>\n      <Description>Collision Energy</Description>\n      <Linked>Fixed</Linked>\n      <Unlinked>Operator</Unlinked>\n      <Location>Compound</Location>\n    </ParaRow>\n    <ParaRow Row=\"19\">\n      <Parameter>CC AF</Parameter>\n      <Channal>10</Channal>\n      <UserMin>-400</UserMin>\n      <UserMax>0</UserMax>\n      <UserDefault>-100</UserDefault>\n      <CalibrationOffset>32768</CalibrationOffset>\n      <CalibrationSlope>-65.8</CalibrationSlope>\n      <ParameterType>7</ParameterType>\n      <Description>Axial Field</Description>\n      <Linked>Fixed</Linked>\n      <Unlinked>Fixed</Unlinked>\n      <Location>Compound</Location>\n    </ParaRow>\n    <ParaRow Row=\"20\">\n      <Parameter>CC L3</Parameter>\n      <Channal>15</Channal>\n      <UserMin>0</UserMin>\n      <UserMax>400</UserMax>\n      <UserDefault>16</UserDefault>\n      <CalibrationOffset>32768</CalibrationOffset>\n      <CalibrationSlope>-65.7</CalibrationSlope>\n      <ParameterType>7</ParameterType>\n      <Description>Collision Cell Lens 3</Description>\n      <Linked>Equation</Linked>\n      <Unlinked>Equation</Unlinked>\n      <Location>Compound</Location>\n    </ParaRow>\n    <ParaRow Row=\"21\">\n      <Parameter>CC L4</Parameter>\n      <Channal>16</Channal>\n      <UserMin>0</UserMin>\n      <UserMax>400</UserMax>\n      <UserDefault>27</UserDefault>\n      <CalibrationOffset>32768</CalibrationOffset>\n      <CalibrationSlope>-65.7</CalibrationSlope>\n      <ParameterType>7</ParameterType>\n      <Description>Collision Cell Lens 4</Description>\n      <Linked>Equation</Linked>\n      <Unlinked>Operator</Unlinked>\n      <Location>Compound</Location>\n    </ParaRow>\n    <ParaRow Row=\"22\">\n      <Parameter>Q2</Parameter>\n      <Channal>8</Channal>\n      <UserMin>0</UserMin>\n      <UserMax>150</UserMax>\n      <UserDefault>17</UserDefault>\n      <CalibrationOffset>32756</CalibrationOffset>\n      <CalibrationSlope>-131.3</CalibrationSlope>\n      <ParameterType>11</ParameterType>\n      <Description>Quadrupole 2</Description>\n      <Linked>Equation</Linked>\n      <Unlinked>Equation</Unlinked>\n      <Location>Resolution</Location>\n    </ParaRow>\n    <ParaRow Row=\"23\">\n      <Parameter>ID</Parameter>\n      <Channal>17</Channal>\n      <UserMin>0</UserMin>\n      <UserMax>400</UserMax>\n      <UserDefault>125</UserDefault>\n      <CalibrationOffset>32768</CalibrationOffset>\n      <CalibrationSlope>-65.8</CalibrationSlope>\n      <ParameterType>7</ParameterType>\n      <Description>Detector Deflector</Description>\n      <Linked>Equation</Linked>\n      <Unlinked>Equation</Unlinked>\n      <Location>Compound</Location>\n    </ParaRow>\n    <ParaRow Row=\"24\">\n      <Parameter>DISC</Parameter>\n      <Channal>32</Channal>\n      <UserMin>10</UserMin>\n      <UserMax>2000</UserMax>\n      <UserDefault>15</UserDefault>\n      <CalibrationOffset>-5</CalibrationOffset>\n      <CalibrationSlope>1.23</CalibrationSlope>\n      <ParameterType>18</ParameterType>\n      <Description>Discriminator</Description>\n      <Linked>Fixed</Linked>\n      <Unlinked>Fixed</Unlinked>\n      <Location>Detector</Location>\n    </ParaRow>\n    <ParaRow Row=\"25\">\n      <Parameter>DV</Parameter>\n      <Channal>34</Channal>\n      <UserMin>1600</UserMin>\n      <UserMax>3500</UserMax>\n      <UserDefault>2000</UserDefault>\n      <CalibrationOffset>0</CalibrationOffset>\n      <CalibrationSlope>0.415</CalibrationSlope>\n      <ParameterType>18</ParameterType>\n      <Description>Detector Voltage</Description>\n      <Linked>Operator</Linked>\n      <Unlinked>Operator</Unlinked>\n      <Location>Detector</Location>\n    </ParaRow>\n    <ParaRow Row=\"26\">\n      <Parameter>DET horn</Parameter>\n      <Channal>200</Channal>\n      <UserMin>0</UserMin>\n      <UserMax>5500</UserMax>\n      <UserDefault>5500</UserDefault>\n      <CalibrationOffset>0</CalibrationOffset>\n      <CalibrationSlope>0.415</CalibrationSlope>\n      <ParameterType>16</ParameterType>\n      <Description>Detector Horn</Description>\n      <Linked>Fixed</Linked>\n      <Unlinked>Fixed</Unlinked>\n      <Location>Detector</Location>\n    </ParaRow>\n    <ParaRow Row=\"27\">\n      <Parameter>LS400A</Parameter>\n      <Channal>36</Channal>\n      <UserMin>0</UserMin>\n      <UserMax>420</UserMax>\n      <UserDefault>420</UserDefault>\n      <CalibrationOffset>0</CalibrationOffset>\n      <CalibrationSlope>8.4</CalibrationSlope>\n      <ParameterType>64</ParameterType>\n      <Description>Lens Power Supply A +400</Description>\n      <Linked>\n      </Linked>\n      <Unlinked>\n      </Unlinked>\n      <Location>\n      </Location>\n    </ParaRow>\n    <ParaRow Row=\"28\">\n      <Parameter>LS-400A</Parameter>\n      <Channal>37</Channal>\n      <UserMin>-420</UserMin>\n      <UserMax>-55</UserMax>\n      <UserDefault>-420</UserDefault>\n      <CalibrationOffset>-433</CalibrationOffset>\n      <CalibrationSlope>-8.4</CalibrationSlope>\n      <ParameterType>64</ParameterType>\n      <Description>Lens Power Supply A -400</Description>\n      <Linked>\n      </Linked>\n      <Unlinked>\n      </Unlinked>\n      <Location>\n      </Location>\n    </ParaRow>\n    <ParaRow Row=\"29\">\n      <Parameter>LS400B</Parameter>\n      <Channal>38</Channal>\n      <UserMin>0</UserMin>\n      <UserMax>420</UserMax>\n      <UserDefault>420</UserDefault>\n      <CalibrationOffset>0</CalibrationOffset>\n      <CalibrationSlope>8.4</CalibrationSlope>\n      <ParameterType>64</ParameterType>\n      <Description>Lens Power Supply B +400</Description>\n      <Linked>\n      </Linked>\n      <Unlinked>\n      </Unlinked>\n      <Location>\n      </Location>\n    </ParaRow>\n    <ParaRow Row=\"30\">\n      <Parameter>LS-400B</Parameter>\n      <Channal>39</Channal>\n      <UserMin>-420</UserMin>\n      <UserMax>-55</UserMax>\n      <UserDefault>-420</UserDefault>\n      <CalibrationOffset>-433</CalibrationOffset>\n      <CalibrationSlope>-8.4</CalibrationSlope>\n      <ParameterType>64</ParameterType>\n      <Description>Lens Power Supply B  -400</Description>\n      <Linked>\n      </Linked>\n      <Unlinked>\n      </Unlinked>\n      <Location>\n      </Location>\n    </ParaRow>\n    <ParaRow Row=\"31\">\n      <Parameter>QPS800</Parameter>\n      <Channal>40</Channal>\n      <UserMin>110</UserMin>\n      <UserMax>600</UserMax>\n      <UserDefault>600</UserDefault>\n      <CalibrationOffset>0</CalibrationOffset>\n      <CalibrationSlope>4.25</CalibrationSlope>\n      <ParameterType>64</ParameterType>\n      <Description>Quad Power Supply +800</Description>\n      <Linked>\n      </Linked>\n      <Unlinked>\n      </Unlinked>\n      <Location>\n      </Location>\n    </ParaRow>\n    <ParaRow Row=\"32\">\n      <Parameter>QPS-800</Parameter>\n      <Channal>41</Channal>\n      <UserMin>-110</UserMin>\n      <UserMax>-110</UserMax>\n      <UserDefault>-600</UserDefault>\n      <CalibrationOffset>-433</CalibrationOffset>\n      <CalibrationSlope>-4.2</CalibrationSlope>\n      <ParameterType>64</ParameterType>\n      <Description>Quad Power Supply -800</Description>\n      <Linked>\n      </Linked>\n      <Unlinked>\n      </Unlinked>\n      <Location>\n      </Location>\n    </ParaRow>\n    <ParaRow Row=\"33\">\n      <Parameter>DG</Parameter>\n      <Channal>26</Channal>\n      <UserMin>50</UserMin>\n      <UserMax>300</UserMax>\n      <UserDefault>80</UserDefault>\n      <CalibrationOffset>0</CalibrationOffset>\n      <CalibrationSlope>32.765</CalibrationSlope>\n      <ParameterType>32</ParameterType>\n      <Description>Drying Gas</Description>\n      <Linked>Operator</Linked>\n      <Unlinked>Operator</Unlinked>\n      <Location>Source</Location>\n    </ParaRow>\n    <ParaRow Row=\"34\">\n      <Parameter>NG1</Parameter>\n      <Channal>27</Channal>\n      <UserMin>0</UserMin>\n      <UserMax>450</UserMax>\n      <UserDefault>0</UserDefault>\n      <CalibrationOffset>0</CalibrationOffset>\n      <CalibrationSlope>32.765</CalibrationSlope>\n      <ParameterType>32</ParameterType>\n      <Description>Nebulizer Gas 1</Description>\n      <Linked>Operator</Linked>\n      <Unlinked>Operator</Unlinked>\n      <Location>Source</Location>\n    </ParaRow>\n    <ParaRow Row=\"35\">\n      <Parameter>HG1</Parameter>\n      <Channal>29</Channal>\n      <UserMin>0</UserMin>\n      <UserMax>350</UserMax>\n      <UserDefault>0</UserDefault>\n      <CalibrationOffset>0</CalibrationOffset>\n      <CalibrationSlope>32.765</CalibrationSlope>\n      <ParameterType>32</ParameterType>\n      <Description>Heating Gas 1</Description>\n      <Linked>Equation</Linked>\n      <Unlinked>Equation</Unlinked>\n      <Location>Source</Location>\n    </ParaRow>\n    <ParaRow Row=\"36\">\n      <Parameter>NG2</Parameter>\n      <Channal>28</Channal>\n      <UserMin>0</UserMin>\n      <UserMax>450</UserMax>\n      <UserDefault>0</UserDefault>\n      <CalibrationOffset>0</CalibrationOffset>\n      <CalibrationSlope>32.765</CalibrationSlope>\n      <ParameterType>32</ParameterType>\n      <Description>Nebulizer Gas 2</Description>\n      <Linked>Operator</Linked>\n      <Unlinked>Operator</Unlinked>\n      <Location>Source</Location>\n    </ParaRow>\n    <ParaRow Row=\"37\">\n      <Parameter>HG2</Parameter>\n      <Channal>30</Channal>\n      <UserMin>0</UserMin>\n      <UserMax>350</UserMax>\n      <UserDefault>0</UserDefault>\n      <CalibrationOffset>0</CalibrationOffset>\n      <CalibrationSlope>32.765</CalibrationSlope>\n      <ParameterType>32</ParameterType>\n      <Description>Heating Gas 2</Description>\n      <Linked>Equation</Linked>\n      <Unlinked>Equation</Unlinked>\n      <Location>Source</Location>\n    </ParaRow>\n    <ParaRow Row=\"38\">\n      <Parameter>CC P</Parameter>\n      <Channal>43</Channal>\n      <UserMin>0</UserMin>\n      <UserMax>500</UserMax>\n      <UserDefault>410</UserDefault>\n      <CalibrationOffset>0</CalibrationOffset>\n      <CalibrationSlope>32.765</CalibrationSlope>\n      <ParameterType>6</ParameterType>\n      <Description>Collision Pressure</Description>\n      <Linked>Fixed</Linked>\n      <Unlinked>Operator</Unlinked>\n      <Location>Compound</Location>\n    </ParaRow>\n    <ParaRow Row=\"39\">\n      <Parameter>SX</Parameter>\n      <Channal>42</Channal>\n      <UserMin>0</UserMin>\n      <UserMax>500</UserMax>\n      <UserDefault>500</UserDefault>\n      <CalibrationOffset>0</CalibrationOffset>\n      <CalibrationSlope>32.765</CalibrationSlope>\n      <ParameterType>32</ParameterType>\n      <Description>Source Exhaust</Description>\n      <Linked>Fixed</Linked>\n      <Unlinked>Fixed</Unlinked>\n      <Location>Source</Location>\n    </ParaRow>\n    <ParaRow Row=\"40\">\n      <Parameter>ISV2</Parameter>\n      <Channal>204</Channal>\n      <UserMin>-5850</UserMin>\n      <UserMax>0</UserMax>\n      <UserDefault>0</UserDefault>\n      <CalibrationOffset>0</CalibrationOffset>\n      <CalibrationSlope>0.0436</CalibrationSlope>\n      <ParameterType>34</ParameterType>\n      <Description>ElectroSpray V2</Description>\n      <Linked>Operator</Linked>\n      <Unlinked>Operator</Unlinked>\n      <Location>Source</Location>\n    </ParaRow>\n    <ParaRow Row=\"41\">\n      <Parameter>ISV1</Parameter>\n      <Channal>203</Channal>\n      <UserMin>-5850</UserMin>\n      <UserMax>0</UserMax>\n      <UserDefault>0</UserDefault>\n      <CalibrationOffset>0</CalibrationOffset>\n      <CalibrationSlope>0.0436</CalibrationSlope>\n      <ParameterType>34</ParameterType>\n      <Description>ElectroSpray V1</Description>\n      <Linked>Operator</Linked>\n      <Unlinked>Operator</Unlinked>\n      <Location>Source</Location>\n    </ParaRow>\n    <ParaRow Row=\"42\">\n      <Parameter>CD</Parameter>\n      <Channal>202</Channal>\n      <UserMin>-5</UserMin>\n      <UserMax>0</UserMax>\n      <UserDefault>0</UserDefault>\n      <CalibrationOffset>0</CalibrationOffset>\n      <CalibrationSlope>51</CalibrationSlope>\n      <ParameterType>34</ParameterType>\n      <Description>Corona Discharge</Description>\n      <Linked>Operator</Linked>\n      <Unlinked>Operator</Unlinked>\n      <Location>Source</Location>\n    </ParaRow>\n    <ParaRow Row=\"43\">\n      <Parameter>CAP</Parameter>\n      <Channal>201</Channal>\n      <UserMin>-1100</UserMin>\n      <UserMax>0</UserMax>\n      <UserDefault>-1000</UserDefault>\n      <CalibrationOffset>0</CalibrationOffset>\n      <CalibrationSlope>0.22</CalibrationSlope>\n      <ParameterType>34</ParameterType>\n      <Description>Curtain Cap</Description>\n      <Linked>Fixed</Linked>\n      <Unlinked>Fixed</Unlinked>\n      <Location>Source</Location>\n    </ParaRow>\n    <ParaRow Row=\"44\">\n      <Parameter>HSID T</Parameter>\n      <Channal>81</Channal>\n      <UserMin>0</UserMin>\n      <UserMax>320</UserMax>\n      <UserDefault>200</UserDefault>\n      <CalibrationOffset>0</CalibrationOffset>\n      <CalibrationSlope>1</CalibrationSlope>\n      <ParameterType>32</ParameterType>\n      <Description>HSID Temperature</Description>\n      <Linked>Operator</Linked>\n      <Unlinked>Operator</Unlinked>\n      <Location>Source</Location>\n    </ParaRow>\n    <ParaRow Row=\"45\">\n      <Parameter>P1 T</Parameter>\n      <Channal>86</Channal>\n      <UserMin>0</UserMin>\n      <UserMax>500</UserMax>\n      <UserDefault>0</UserDefault>\n      <CalibrationOffset>0</CalibrationOffset>\n      <CalibrationSlope>1</CalibrationSlope>\n      <ParameterType>32</ParameterType>\n      <Description>Source 1 Temp</Description>\n      <Linked>Operator</Linked>\n      <Unlinked>Operator</Unlinked>\n      <Location>Source</Location>\n    </ParaRow>\n    <ParaRow Row=\"46\">\n      <Parameter>P2 T</Parameter>\n      <Channal>84</Channal>\n      <UserMin>0</UserMin>\n      <UserMax>500</UserMax>\n      <UserDefault>0</UserDefault>\n      <CalibrationOffset>0</CalibrationOffset>\n      <CalibrationSlope>1</CalibrationSlope>\n      <ParameterType>32</ParameterType>\n      <Description>Source 2 Temp</Description>\n      <Linked>Operator</Linked>\n      <Unlinked>Operator</Unlinked>\n      <Location>Source</Location>\n    </ParaRow>\n  </ScanType>", "<ScanType name=\"MS/MSPositive\">\n    <ParaRow Row=\"1\">\n      <Parameter>Q1 RF</Parameter>\n      <Channal>1</Channal>\n      <UserMin>10</UserMin>\n      <UserMax>2150</UserMax>\n      <UserDefault>400</UserDefault>\n      <CalibrationOffset>0</CalibrationOffset>\n      <CalibrationSlope>218.45</CalibrationSlope>\n      <ParameterType>64</ParameterType>\n      <Description>Quadrupole 1 RF</Description>\n      <Linked>\n      </Linked>\n      <Unlinked>\n      </Unlinked>\n      <Location>\n      </Location>\n    </ParaRow>\n    <ParaRow Row=\"2\">\n      <Parameter>Q1 DC</Parameter>\n      <Channal>4</Channal>\n      <UserMin>10</UserMin>\n      <UserMax>2150</UserMax>\n      <UserDefault>600</UserDefault>\n      <CalibrationOffset>0</CalibrationOffset>\n      <CalibrationSlope>218.45</CalibrationSlope>\n      <ParameterType>64</ParameterType>\n      <Description>Quadrupole 1 DC</Description>\n      <Linked>\n      </Linked>\n      <Unlinked>\n      </Unlinked>\n      <Location>\n      </Location>\n    </ParaRow>\n    <ParaRow Row=\"3\">\n      <Parameter>Q1 RR</Parameter>\n      <Channal>7</Channal>\n      <UserMin>0</UserMin>\n      <UserMax>64000</UserMax>\n      <UserDefault>32768</UserDefault>\n      <CalibrationOffset>32768</CalibrationOffset>\n      <CalibrationSlope>1</CalibrationSlope>\n      <ParameterType>64</ParameterType>\n      <Description>Quadrupole 1 PW</Description>\n      <Linked>\n      </Linked>\n      <Unlinked>\n      </Unlinked>\n      <Location>\n      </Location>\n    </ParaRow>\n    <ParaRow Row=\"4\">\n      <Parameter>Q2 RF</Parameter>\n      <Channal>2</Channal>\n      <UserMin>10</UserMin>\n      <UserMax>2150</UserMax>\n      <UserDefault>400</UserDefault>\n      <CalibrationOffset>0</CalibrationOffset>\n      <CalibrationSlope>218.45</CalibrationSlope>\n      <ParameterType>64</ParameterType>\n      <Description>Quadrupole 2 RF</Description>\n      <Linked>\n      </Linked>\n      <Unlinked>\n      </Unlinked>\n      <Location>\n      </Location>\n    </ParaRow>\n    <ParaRow Row=\"5\">\n      <Parameter>Q2 DC</Parameter>\n      <Channal>5</Channal>\n      <UserMin>10</UserMin>\n      <UserMax>2150</UserMax>\n      <UserDefault>600</UserDefault>\n      <CalibrationOffset>0</CalibrationOffset>\n      <CalibrationSlope>218.45</CalibrationSlope>\n      <ParameterType>64</ParameterType>\n      <Description>Quadrupole 2 DC</Description>\n      <Linked>\n      </Linked>\n      <Unlinked>\n      </Unlinked>\n      <Location>\n      </Location>\n    </ParaRow>\n    <ParaRow Row=\"6\">\n      <Parameter>Q2 RR</Parameter>\n      <Channal>9</Channal>\n      <UserMin>0</UserMin>\n      <UserMax>64000</UserMax>\n      <UserDefault>32768</UserDefault>\n      <CalibrationOffset>32768</CalibrationOffset>\n      <CalibrationSlope>1</CalibrationSlope>\n      <ParameterType>64</ParameterType>\n      <Description>Quadrupole 2 PW</Description>\n      <Linked>\n      </Linked>\n      <Unlinked>\n      </Unlinked>\n      <Location>\n      </Location>\n    </ParaRow>\n    <ParaRow Row=\"7\">\n      <Parameter>M1 RF</Parameter>\n      <Channal>3</Channal>\n      <UserMin>0</UserMin>\n      <UserMax>600</UserMax>\n      <UserDefault>500</UserDefault>\n      <CalibrationOffset>0</CalibrationOffset>\n      <CalibrationSlope>14.7</CalibrationSlope>\n      <ParameterType>6</ParameterType>\n      <Description>Multipole 1 RF</Description>\n      <Linked>Fixed</Linked>\n      <Unlinked>Operator</Unlinked>\n      <Location>Compound</Location>\n    </ParaRow>\n    <ParaRow Row=\"8\">\n      <Parameter>EV</Parameter>\n      <Channal>20</Channal>\n      <UserMin>0</UserMin>\n      <UserMax>200</UserMax>\n      <UserDefault>100</UserDefault>\n      <CalibrationOffset>32768</CalibrationOffset>\n      <CalibrationSlope>-65.7</CalibrationSlope>\n      <ParameterType>7</ParameterType>\n      <Description>Entrance Voltage</Description>\n      <Linked>Operator</Linked>\n      <Unlinked>Operator</Unlinked>\n      <Location>Compound</Location>\n    </ParaRow>\n    <ParaRow Row=\"9\">\n      <Parameter>ED</Parameter>\n      <Channal>21</Channal>\n      <UserMin>0</UserMin>\n      <UserMax>200</UserMax>\n      <UserDefault>90</UserDefault>\n      <CalibrationOffset>32768</CalibrationOffset>\n      <CalibrationSlope>-65.5</CalibrationSlope>\n      <ParameterType>7</ParameterType>\n      <Description>Entrance Deflector</Description>\n      <Linked>Operator</Linked>\n      <Unlinked>Operator</Unlinked>\n      <Location>Compound</Location>\n    </ParaRow>\n    <ParaRow Row=\"10\">\n      <Parameter>M1</Parameter>\n      <Channal>19</Channal>\n      <UserMin>-10</UserMin>\n      <UserMax>5</UserMax>\n      <UserDefault>-1</UserDefault>\n      <CalibrationOffset>32768</CalibrationOffset>\n      <CalibrationSlope>-65.6</CalibrationSlope>\n      <ParameterType>7</ParameterType>\n      <Description>Multipole 1</Description>\n      <Linked>Equation</Linked>\n      <Unlinked>Equation</Unlinked>\n      <Location>Compound</Location>\n    </ParaRow>\n    <ParaRow Row=\"11\">\n      <Parameter>L1</Parameter>\n      <Channal>18</Channal>\n      <UserMin>-10</UserMin>\n      <UserMax>5</UserMax>\n      <UserDefault>-2</UserDefault>\n      <CalibrationOffset>32760</CalibrationOffset>\n      <CalibrationSlope>-65.9</CalibrationSlope>\n      <ParameterType>7</ParameterType>\n      <Description>Multipole Lens 1</Description>\n      <Linked>Equation</Linked>\n      <Unlinked>Equation</Unlinked>\n      <Location>Compound</Location>\n    </ParaRow>\n    <ParaRow Row=\"12\">\n      <Parameter>M2</Parameter>\n      <Channal>22</Channal>\n      <UserMin>-10</UserMin>\n      <UserMax>5</UserMax>\n      <UserDefault>-3</UserDefault>\n      <CalibrationOffset>32768</CalibrationOffset>\n      <CalibrationSlope>-66</CalibrationSlope>\n      <ParameterType>7</ParameterType>\n      <Description>Multipole 2</Description>\n      <Linked>Fixed</Linked>\n      <Unlinked>Fixed</Unlinked>\n      <Location>Compound</Location>\n    </ParaRow>\n    <ParaRow Row=\"13\">\n      <Parameter>L2</Parameter>\n      <Channal>11</Channal>\n      <UserMin>-10</UserMin>\n      <UserMax>5</UserMax>\n      <UserDefault>-4</UserDefault>\n      <CalibrationOffset>32768</CalibrationOffset>\n      <CalibrationSlope>-65.9</CalibrationSlope>\n      <ParameterType>7</ParameterType>\n      <Description>Multipole Lens 2</Description>\n      <Linked>Equation</Linked>\n      <Unlinked>Equation</Unlinked>\n      <Location>Compound</Location>\n    </ParaRow>\n    <ParaRow Row=\"14\">\n      <Parameter>PF</Parameter>\n      <Channal>12</Channal>\n      <UserMin>-50</UserMin>\n      <UserMax>5</UserMax>\n      <UserDefault>-15</UserDefault>\n      <CalibrationOffset>32768</CalibrationOffset>\n      <CalibrationSlope>-65.8</CalibrationSlope>\n      <ParameterType>7</ParameterType>\n      <Description>Prefilter 1</Description>\n      <Linked>Equation</Linked>\n      <Unlinked>Operator</Unlinked>\n      <Location>Compound</Location>\n    </ParaRow>\n    <ParaRow Row=\"15\">\n      <Parameter>Q1</Parameter>\n      <Channal>6</Channal>\n      <UserMin>-10</UserMin>\n      <UserMax>0</UserMax>\n      <UserDefault>-4.5</UserDefault>\n      <CalibrationOffset>32755</CalibrationOffset>\n      <CalibrationSlope>-131.3</CalibrationSlope>\n      <ParameterType>11</ParameterType>\n      <Description>Quadrupole 1</Description>\n      <Linked>Equation</Linked>\n      <Unlinked>Equation</Unlinked>\n      <Location>Resolution</Location>\n    </ParaRow>\n    <ParaRow Row=\"16\">\n      <Parameter>CC L1</Parameter>\n      <Channal>13</Channal>\n      <UserMin>-100</UserMin>\n      <UserMax>10</UserMax>\n      <UserDefault>-10</UserDefault>\n      <CalibrationOffset>32768</CalibrationOffset>\n      <CalibrationSlope>-65.8</CalibrationSlope>\n      <ParameterType>7</ParameterType>\n      <Description>Collision Cell Lens 1</Description>\n      <Linked>Equation</Linked>\n      <Unlinked>Operator</Unlinked>\n      <Location>Compound</Location>\n    </ParaRow>\n    <ParaRow Row=\"17\">\n      <Parameter>CC L2</Parameter>\n      <Channal>14</Channal>\n      <UserMin>-400</UserMin>\n      <UserMax>0</UserMax>\n      <UserDefault>-100</UserDefault>\n      <CalibrationOffset>32768</CalibrationOffset>\n      <CalibrationSlope>-65.8</CalibrationSlope>\n      <ParameterType>7</ParameterType>\n      <Description>Collision Cell Lens 2</Description>\n      <Linked>Operator</Linked>\n      <Unlinked>Operator</Unlinked>\n      <Location>Compound</Location>\n    </ParaRow>\n    <ParaRow Row=\"18\">\n      <Parameter>CC</Parameter>\n      <Channal>23</Channal>\n      <UserMin>-150</UserMin>\n      <UserMax>0</UserMax>\n      <UserDefault>-50</UserDefault>\n      <CalibrationOffset>32768</CalibrationOffset>\n      <CalibrationSlope>-65.8</CalibrationSlope>\n      <ParameterType>7</ParameterType>\n      <Description>Collision Energy</Description>\n      <Linked>Operator</Linked>\n      <Unlinked>Operator</Unlinked>\n      <Location>Compound</Location>\n    </ParaRow>\n    <ParaRow Row=\"19\">\n      <Parameter>CC AF</Parameter>\n      <Channal>10</Channal>\n      <UserMin>0</UserMin>\n      <UserMax>400</UserMax>\n      <UserDefault>100</UserDefault>\n      <CalibrationOffset>32768</CalibrationOffset>\n      <CalibrationSlope>-65.8</CalibrationSlope>\n      <ParameterType>7</ParameterType>\n      <Description>Axial Field</Description>\n      <Linked>Fixed</Linked>\n      <Unlinked>Operator</Unlinked>\n      <Location>Compound</Location>\n    </ParaRow>\n    <ParaRow Row=\"20\">\n      <Parameter>CC L3</Parameter>\n      <Channal>15</Channal>\n      <UserMin>-200</UserMin>\n      <UserMax>0</UserMax>\n      <UserDefault>-51</UserDefault>\n      <CalibrationOffset>32768</CalibrationOffset>\n      <CalibrationSlope>-65.7</CalibrationSlope>\n      <ParameterType>7</ParameterType>\n      <Description>Collision Cell Lens 3</Description>\n      <Linked>Equation</Linked>\n      <Unlinked>Equation</Unlinked>\n      <Location>Compound</Location>\n    </ParaRow>\n    <ParaRow Row=\"21\">\n      <Parameter>CC L4</Parameter>\n      <Channal>16</Channal>\n      <UserMin>-400</UserMin>\n      <UserMax>0</UserMax>\n      <UserDefault>-62</UserDefault>\n      <CalibrationOffset>32768</CalibrationOffset>\n      <CalibrationSlope>-65.7</CalibrationSlope>\n      <ParameterType>7</ParameterType>\n      <Description>Collision Cell Lens 4</Description>\n      <Linked>Equation</Linked>\n      <Unlinked>Equation</Unlinked>\n      <Location>Compound</Location>\n    </ParaRow>\n    <ParaRow Row=\"22\">\n      <Parameter>Q2</Parameter>\n      <Channal>8</Channal>\n      <UserMin>-150</UserMin>\n      <UserMax>0</UserMax>\n      <UserDefault>-52</UserDefault>\n      <CalibrationOffset>32756</CalibrationOffset>\n      <CalibrationSlope>-131.3</CalibrationSlope>\n      <ParameterType>11</ParameterType>\n      <Description>Quadrupole 2</Description>\n      <Linked>Equation</Linked>\n      <Unlinked>Equation</Unlinked>\n      <Location>Resolution</Location>\n    </ParaRow>\n    <ParaRow Row=\"23\">\n      <Parameter>ID</Parameter>\n      <Channal>17</Channal>\n      <UserMin>-400</UserMin>\n      <UserMax>0</UserMax>\n      <UserDefault>-140</UserDefault>\n      <CalibrationOffset>32768</CalibrationOffset>\n      <CalibrationSlope>-65.8</CalibrationSlope>\n      <ParameterType>7</ParameterType>\n      <Description>Detector Deflector</Description>\n      <Linked>Equation</Linked>\n      <Unlinked>Operator</Unlinked>\n      <Location>Compound</Location>\n    </ParaRow>\n    <ParaRow Row=\"24\">\n      <Parameter>DISC</Parameter>\n      <Channal>32</Channal>\n      <UserMin>10</UserMin>\n      <UserMax>2000</UserMax>\n      <UserDefault>15</UserDefault>\n      <CalibrationOffset>-5</CalibrationOffset>\n      <CalibrationSlope>1.23</CalibrationSlope>\n      <ParameterType>18</ParameterType>\n      <Description>Discriminator</Description>\n      <Linked>Fixed</Linked>\n      <Unlinked>Fixed</Unlinked>\n      <Location>Detector</Location>\n    </ParaRow>\n    <ParaRow Row=\"25\">\n      <Parameter>DV</Parameter>\n      <Channal>34</Channal>\n      <UserMin>1600</UserMin>\n      <UserMax>3500</UserMax>\n      <UserDefault>2000</UserDefault>\n      <CalibrationOffset>0</CalibrationOffset>\n      <CalibrationSlope>0.415</CalibrationSlope>\n      <ParameterType>18</ParameterType>\n      <Description>Detector Voltage</Description>\n      <Linked>Operator</Linked>\n      <Unlinked>Operator</Unlinked>\n      <Location>Detector</Location>\n    </ParaRow>\n    <ParaRow Row=\"26\">\n      <Parameter>DET horn</Parameter>\n      <Channal>200</Channal>\n      <UserMin>0</UserMin>\n      <UserMax>5500</UserMax>\n      <UserDefault>5500</UserDefault>\n      <CalibrationOffset>0</CalibrationOffset>\n      <CalibrationSlope>0.415</CalibrationSlope>\n      <ParameterType>16</ParameterType>\n      <Description>Detector Horn</Description>\n      <Linked>Fixed</Linked>\n      <Unlinked>Fixed</Unlinked>\n      <Location>Detector</Location>\n    </ParaRow>\n    <ParaRow Row=\"27\">\n      <Parameter>LS400A</Parameter>\n      <Channal>36</Channal>\n      <UserMin>0</UserMin>\n      <UserMax>420</UserMax>\n      <UserDefault>420</UserDefault>\n      <CalibrationOffset>0</CalibrationOffset>\n      <CalibrationSlope>8.4</CalibrationSlope>\n      <ParameterType>64</ParameterType>\n      <Description>Lens Power Supply A +400</Description>\n      <Linked>\n      </Linked>\n      <Unlinked>\n      </Unlinked>\n      <Location>\n      </Location>\n    </ParaRow>\n    <ParaRow Row=\"28\">\n      <Parameter>LS-400A</Parameter>\n      <Channal>37</Channal>\n      <UserMin>-420</UserMin>\n      <UserMax>-55</UserMax>\n      <UserDefault>-420</UserDefault>\n      <CalibrationOffset>-433</CalibrationOffset>\n      <CalibrationSlope>-8.4</CalibrationSlope>\n      <ParameterType>64</ParameterType>\n      <Description>Lens Power Supply A -400</Description>\n      <Linked>\n      </Linked>\n      <Unlinked>\n      </Unlinked>\n      <Location>\n      </Location>\n    </ParaRow>\n    <ParaRow Row=\"29\">\n      <Parameter>LS400B</Parameter>\n      <Channal>38</Channal>\n      <UserMin>0</UserMin>\n      <UserMax>420</UserMax>\n      <UserDefault>420</UserDefault>\n      <CalibrationOffset>0</CalibrationOffset>\n      <CalibrationSlope>8.4</CalibrationSlope>\n      <ParameterType>64</ParameterType>\n      <Description>Lens Power Supply B +400</Description>\n      <Linked>\n      </Linked>\n      <Unlinked>\n      </Unlinked>\n      <Location>\n      </Location>\n    </ParaRow>\n    <ParaRow Row=\"30\">\n      <Parameter>LS-400B</Parameter>\n      <Channal>39</Channal>\n      <UserMin>-420</UserMin>\n      <UserMax>-55</UserMax>\n      <UserDefault>-420</UserDefault>\n      <CalibrationOffset>-433</CalibrationOffset>\n      <CalibrationSlope>-8.4</CalibrationSlope>\n      <ParameterType>64</ParameterType>\n      <Description>Lens Power Supply B  -400</Description>\n      <Linked>\n      </Linked>\n      <Unlinked>\n      </Unlinked>\n      <Location>\n      </Location>\n    </ParaRow>\n    <ParaRow Row=\"31\">\n      <Parameter>QPS800</Parameter>\n      <Channal>40</Channal>\n      <UserMin>110</UserMin>\n      <UserMax>600</UserMax>\n      <UserDefault>600</UserDefault>\n      <CalibrationOffset>0</CalibrationOffset>\n      <CalibrationSlope>4.25</CalibrationSlope>\n      <ParameterType>64</ParameterType>\n      <Description>Quad Power Supply +800</Description>\n      <Linked>\n      </Linked>\n      <Unlinked>\n      </Unlinked>\n      <Location>\n      </Location>\n    </ParaRow>\n    <ParaRow Row=\"32\">\n      <Parameter>QPS-800</Parameter>\n      <Channal>41</Channal>\n      <UserMin>-110</UserMin>\n      <UserMax>-110</UserMax>\n      <UserDefault>-600</UserDefault>\n      <CalibrationOffset>-433</CalibrationOffset>\n      <CalibrationSlope>-4.2</CalibrationSlope>\n      <ParameterType>64</ParameterType>\n      <Description>Quad Power Supply -800</Description>\n      <Linked>\n      </Linked>\n      <Unlinked>\n      </Unlinked>\n      <Location>\n      </Location>\n    </ParaRow>\n    <ParaRow Row=\"33\">\n      <Parameter>DG</Parameter>\n      <Channal>26</Channal>\n      <UserMin>50</UserMin>\n      <UserMax>200</UserMax>\n      <UserDefault>80</UserDefault>\n      <CalibrationOffset>0</CalibrationOffset>\n      <CalibrationSlope>32.765</CalibrationSlope>\n      <ParameterType>32</ParameterType>\n      <Description>Drying Gas</Description>\n      <Linked>Operator</Linked>\n      <Unlinked>Operator</Unlinked>\n      <Location>Source</Location>\n    </ParaRow>\n    <ParaRow Row=\"34\">\n      <Parameter>NG1</Parameter>\n      <Channal>27</Channal>\n      <UserMin>0</UserMin>\n      <UserMax>450</UserMax>\n      <UserDefault>0</UserDefault>\n      <CalibrationOffset>0</CalibrationOffset>\n      <CalibrationSlope>32.765</CalibrationSlope>\n      <ParameterType>32</ParameterType>\n      <Description>Nebulizer Gas 1</Description>\n      <Linked>Operator</Linked>\n      <Unlinked>Operator</Unlinked>\n      <Location>Source</Location>\n    </ParaRow>\n    <ParaRow Row=\"35\">\n      <Parameter>HG1</Parameter>\n      <Channal>29</Channal>\n      <UserMin>0</UserMin>\n      <UserMax>350</UserMax>\n      <UserDefault>0</UserDefault>\n      <CalibrationOffset>0</CalibrationOffset>\n      <CalibrationSlope>32.765</CalibrationSlope>\n      <ParameterType>32</ParameterType>\n      <Description>Heating Gas 1</Description>\n      <Linked>Equation</Linked>\n      <Unlinked>Equation</Unlinked>\n      <Location>Source</Location>\n    </ParaRow>\n    <ParaRow Row=\"36\">\n      <Parameter>NG2</Parameter>\n      <Channal>28</Channal>\n      <UserMin>0</UserMin>\n      <UserMax>450</UserMax>\n      <UserDefault>0</UserDefault>\n      <CalibrationOffset>0</CalibrationOffset>\n      <CalibrationSlope>32.765</CalibrationSlope>\n      <ParameterType>32</ParameterType>\n      <Description>Nebulizer Gas 2</Description>\n      <Linked>Operator</Linked>\n      <Unlinked>Operator</Unlinked>\n      <Location>Source</Location>\n    </ParaRow>\n    <ParaRow Row=\"37\">\n      <Parameter>HG2</Parameter>\n      <Channal>30</Channal>\n      <UserMin>0</UserMin>\n      <UserMax>350</UserMax>\n      <UserDefault>0</UserDefault>\n      <CalibrationOffset>0</CalibrationOffset>\n      <CalibrationSlope>32.765</CalibrationSlope>\n      <ParameterType>32</ParameterType>\n      <Description>Heating Gas 2</Description>\n      <Linked>Equation</Linked>\n      <Unlinked>Equation</Unlinked>\n      <Location>Source</Location>\n    </ParaRow>\n    <ParaRow Row=\"38\">\n      <Parameter>CC P</Parameter>\n      <Channal>43</Channal>\n      <UserMin>0</UserMin>\n      <UserMax>500</UserMax>\n      <UserDefault>410</UserDefault>\n      <CalibrationOffset>0</CalibrationOffset>\n      <CalibrationSlope>32.765</CalibrationSlope>\n      <ParameterType>6</ParameterType>\n      <Description>Collision Pressure</Description>\n      <Linked>Fixed</Linked>\n      <Unlinked>Operator</Unlinked>\n      <Location>Compound</Location>\n    </ParaRow>\n    <ParaRow Row=\"39\">\n      <Parameter>SX</Parameter>\n      <Channal>42</Channal>\n      <UserMin>0</UserMin>\n      <UserMax>500</UserMax>\n      <UserDefault>500</UserDefault>\n      <CalibrationOffset>0</CalibrationOffset>\n      <CalibrationSlope>32.765</CalibrationSlope>\n      <ParameterType>32</ParameterType>\n      <Description>Source Exhaust</Description>\n      <Linked>Fixed</Linked>\n      <Unlinked>Fixed</Unlinked>\n      <Location>Source</Location>\n    </ParaRow>\n    <ParaRow Row=\"40\">\n      <Parameter>ISV2</Parameter>\n      <Channal>204</Channal>\n      <UserMin>0</UserMin>\n      <UserMax>5850</UserMax>\n      <UserDefault>0</UserDefault>\n      <CalibrationOffset>0</CalibrationOffset>\n      <CalibrationSlope>0.0436</CalibrationSlope>\n      <ParameterType>34</ParameterType>\n      <Description>ElectroSpray V2</Description>\n      <Linked>Operator</Linked>\n      <Unlinked>Operator</Unlinked>\n      <Location>Source</Location>\n    </ParaRow>\n    <ParaRow Row=\"41\">\n      <Parameter>ISV1</Parameter>\n      <Channal>203</Channal>\n      <UserMin>0</UserMin>\n      <UserMax>5850</UserMax>\n      <UserDefault>0</UserDefault>\n      <CalibrationOffset>0</CalibrationOffset>\n      <CalibrationSlope>0.0436</CalibrationSlope>\n      <ParameterType>34</ParameterType>\n      <Description>ElectroSpray V1</Description>\n      <Linked>Operator</Linked>\n      <Unlinked>Operator</Unlinked>\n      <Location>Source</Location>\n    </ParaRow>\n    <ParaRow Row=\"42\">\n      <Parameter>CD</Parameter>\n      <Channal>202</Channal>\n      <UserMin>0</UserMin>\n      <UserMax>5</UserMax>\n      <UserDefault>0</UserDefault>\n      <CalibrationOffset>0</CalibrationOffset>\n      <CalibrationSlope>51</CalibrationSlope>\n      <ParameterType>34</ParameterType>\n      <Description>Corona Discharge</Description>\n      <Linked>Operator</Linked>\n      <Unlinked>Operator</Unlinked>\n      <Location>Source</Location>\n    </ParaRow>\n    <ParaRow Row=\"43\">\n      <Parameter>CAP</Parameter>\n      <Channal>201</Channal>\n      <UserMin>0</UserMin>\n      <UserMax>1100</UserMax>\n      <UserDefault>1000</UserDefault>\n      <CalibrationOffset>0</CalibrationOffset>\n      <CalibrationSlope>0.22</CalibrationSlope>\n      <ParameterType>34</ParameterType>\n      <Description>Curtain Cap</Description>\n      <Linked>Fixed</Linked>\n      <Unlinked>Fixed</Unlinked>\n      <Location>Source</Location>\n    </ParaRow>\n    <ParaRow Row=\"44\">\n      <Parameter>HSID T</Parameter>\n      <Channal>81</Channal>\n      <UserMin>0</UserMin>\n      <UserMax>320</UserMax>\n      <UserDefault>200</UserDefault>\n      <CalibrationOffset>0</CalibrationOffset>\n      <CalibrationSlope>1</CalibrationSlope>\n      <ParameterType>32</ParameterType>\n      <Description>HSID Temperature</Description>\n      <Linked>Operator</Linked>\n      <Unlinked>Operator</Unlinked>\n      <Location>Source</Location>\n    </ParaRow>\n    <ParaRow Row=\"45\">\n      <Parameter>P1 T</Parameter>\n      <Channal>86</Channal>\n      <UserMin>0</UserMin>\n      <UserMax>500</UserMax>\n      <UserDefault>0</UserDefault>\n      <CalibrationOffset>0</CalibrationOffset>\n      <CalibrationSlope>1</CalibrationSlope>\n      <ParameterType>32</ParameterType>\n      <Description>Source 1 Temp</Description>\n      <Linked>Operator</Linked>\n      <Unlinked>Operator</Unlinked>\n      <Location>Source</Location>\n    </ParaRow>\n    <ParaRow Row=\"46\">\n      <Parameter>P2 T</Parameter>\n      <Channal>84</Channal>\n      <UserMin>0</UserMin>\n      <UserMax>500</UserMax>\n      <UserDefault>0</UserDefault>\n      <CalibrationOffset>0</CalibrationOffset>\n      <CalibrationSlope>1</CalibrationSlope>\n      <ParameterType>32</ParameterType>\n      <Description>Source 2 Temp</Description>\n      <Linked>Operator</Linked>\n      <Unlinked>Operator</Unlinked>\n      <Location>Source</Location>\n    </ParaRow>\n  </ScanType>", "<ScanType name=\"MS/MSNegative\">\n    <ParaRow Row=\"1\">\n      <Parameter>Q1 RF</Parameter>\n      <Channal>1</Channal>\n      <UserMin>10</UserMin>\n      <UserMax>2150</UserMax>\n      <UserDefault>400</UserDefault>\n      <CalibrationOffset>0</CalibrationOffset>\n      <CalibrationSlope>218.45</CalibrationSlope>\n      <ParameterType>64</ParameterType>\n      <Description>Quadrupole 1 RF</Description>\n      <Linked>\n      </Linked>\n      <Unlinked>\n      </Unlinked>\n      <Location>\n      </Location>\n    </ParaRow>\n    <ParaRow Row=\"2\">\n      <Parameter>Q1 DC</Parameter>\n      <Channal>4</Channal>\n      <UserMin>10</UserMin>\n      <UserMax>2150</UserMax>\n      <UserDefault>600</UserDefault>\n      <CalibrationOffset>0</CalibrationOffset>\n      <CalibrationSlope>218.45</CalibrationSlope>\n      <ParameterType>64</ParameterType>\n      <Description>Quadrupole 1 DC</Description>\n      <Linked>\n      </Linked>\n      <Unlinked>\n      </Unlinked>\n      <Location>\n      </Location>\n    </ParaRow>\n    <ParaRow Row=\"3\">\n      <Parameter>Q1 RR</Parameter>\n      <Channal>7</Channal>\n      <UserMin>0</UserMin>\n      <UserMax>64000</UserMax>\n      <UserDefault>32768</UserDefault>\n      <CalibrationOffset>32768</CalibrationOffset>\n      <CalibrationSlope>1</CalibrationSlope>\n      <ParameterType>64</ParameterType>\n      <Description>Quadrupole 1 PW</Description>\n      <Linked>\n      </Linked>\n      <Unlinked>\n      </Unlinked>\n      <Location>\n      </Location>\n    </ParaRow>\n    <ParaRow Row=\"4\">\n      <Parameter>Q2 RF</Parameter>\n      <Channal>2</Channal>\n      <UserMin>10</UserMin>\n      <UserMax>2150</UserMax>\n      <UserDefault>400</UserDefault>\n      <CalibrationOffset>0</CalibrationOffset>\n      <CalibrationSlope>218.45</CalibrationSlope>\n      <ParameterType>64</ParameterType>\n      <Description>Quadrupole 2 RF</Description>\n      <Linked>\n      </Linked>\n      <Unlinked>\n      </Unlinked>\n      <Location>\n      </Location>\n    </ParaRow>\n    <ParaRow Row=\"5\">\n      <Parameter>Q2 DC</Parameter>\n      <Channal>5</Channal>\n      <UserMin>10</UserMin>\n      <UserMax>2150</UserMax>\n      <UserDefault>600</UserDefault>\n      <CalibrationOffset>0</CalibrationOffset>\n      <CalibrationSlope>218.45</CalibrationSlope>\n      <ParameterType>64</ParameterType>\n      <Description>Quadrupole 2 DC</Description>\n      <Linked>\n      </Linked>\n      <Unlinked>\n      </Unlinked>\n      <Location>\n      </Location>\n    </ParaRow>\n    <ParaRow Row=\"6\">\n      <Parameter>Q2 RR</Parameter>\n      <Channal>9</Channal>\n      <UserMin>0</UserMin>\n      <UserMax>64000</UserMax>\n      <UserDefault>32768</UserDefault>\n      <CalibrationOffset>32768</CalibrationOffset>\n      <CalibrationSlope>1</CalibrationSlope>\n      <ParameterType>64</ParameterType>\n      <Description>Quadrupole 2 PW</Description>\n      <Linked>\n      </Linked>\n      <Unlinked>\n      </Unlinked>\n      <Location>\n      </Location>\n    </ParaRow>\n    <ParaRow Row=\"7\">\n      <Parameter>M1 RF</Parameter>\n      <Channal>3</Channal>\n      <UserMin>0</UserMin>\n      <UserMax>600</UserMax>\n      <UserDefault>500</UserDefault>\n      <CalibrationOffset>0</CalibrationOffset>\n      <CalibrationSlope>14.7</CalibrationSlope>\n      <ParameterType>6</ParameterType>\n      <Description>Multipole 1 RF</Description>\n      <Linked>Fixed</Linked>\n      <Unlinked>Operator</Unlinked>\n      <Location>Compound</Location>\n    </ParaRow>\n    <ParaRow Row=\"8\">\n      <Parameter>EV</Parameter>\n      <Channal>20</Channal>\n      <UserMin>-200</UserMin>\n      <UserMax>0</UserMax>\n      <UserDefault>-100</UserDefault>\n      <CalibrationOffset>32768</CalibrationOffset>\n      <CalibrationSlope>-65.7</CalibrationSlope>\n      <ParameterType>7</ParameterType>\n      <Description>Entrance Voltage</Description>\n      <Linked>Operator</Linked>\n      <Unlinked>Operator</Unlinked>\n      <Location>Compound</Location>\n    </ParaRow>\n    <ParaRow Row=\"9\">\n      <Parameter>ED</Parameter>\n      <Channal>21</Channal>\n      <UserMin>-200</UserMin>\n      <UserMax>0</UserMax>\n      <UserDefault>-90</UserDefault>\n      <CalibrationOffset>32768</CalibrationOffset>\n      <CalibrationSlope>-65.5</CalibrationSlope>\n      <ParameterType>7</ParameterType>\n      <Description>Entrance Deflector</Description>\n      <Linked>Operator</Linked>\n      <Unlinked>Operator</Unlinked>\n      <Location>Compound</Location>\n    </ParaRow>\n    <ParaRow Row=\"10\">\n      <Parameter>M1</Parameter>\n      <Channal>19</Channal>\n      <UserMin>-5</UserMin>\n      <UserMax>10</UserMax>\n      <UserDefault>1</UserDefault>\n      <CalibrationOffset>32768</CalibrationOffset>\n      <CalibrationSlope>-65.6</CalibrationSlope>\n      <ParameterType>7</ParameterType>\n      <Description>Multipole 1</Description>\n      <Linked>Equation</Linked>\n      <Unlinked>Equation</Unlinked>\n      <Location>Compound</Location>\n    </ParaRow>\n    <ParaRow Row=\"11\">\n      <Parameter>L1</Parameter>\n      <Channal>18</Channal>\n      <UserMin>-5</UserMin>\n      <UserMax>10</UserMax>\n      <UserDefault>2</UserDefault>\n      <CalibrationOffset>32760</CalibrationOffset>\n      <CalibrationSlope>-65.9</CalibrationSlope>\n      <ParameterType>7</ParameterType>\n      <Description>Multipole Lens 1</Description>\n      <Linked>Equation</Linked>\n      <Unlinked>Equation</Unlinked>\n      <Location>Compound</Location>\n    </ParaRow>\n    <ParaRow Row=\"12\">\n      <Parameter>M2</Parameter>\n      <Channal>22</Channal>\n      <UserMin>-5</UserMin>\n      <UserMax>10</UserMax>\n      <UserDefault>3</UserDefault>\n      <CalibrationOffset>32768</CalibrationOffset>\n      <CalibrationSlope>-66</CalibrationSlope>\n      <ParameterType>7</ParameterType>\n      <Description>Multipole 2</Description>\n      <Linked>Fixed</Linked>\n      <Unlinked>Fixed</Unlinked>\n      <Location>Compound</Location>\n    </ParaRow>\n    <ParaRow Row=\"13\">\n      <Parameter>L2</Parameter>\n      <Channal>11</Channal>\n      <UserMin>-5</UserMin>\n      <UserMax>10</UserMax>\n      <UserDefault>4</UserDefault>\n      <CalibrationOffset>32768</CalibrationOffset>\n      <CalibrationSlope>-65.9</CalibrationSlope>\n      <ParameterType>7</ParameterType>\n      <Description>Multipole Lens 2</Description>\n      <Linked>Equation</Linked>\n      <Unlinked>Equation</Unlinked>\n      <Location>Compound</Location>\n    </ParaRow>\n    <ParaRow Row=\"14\">\n      <Parameter>PF</Parameter>\n      <Channal>12</Channal>\n      <UserMin>-5</UserMin>\n      <UserMax>50</UserMax>\n      <UserDefault>15</UserDefault>\n      <CalibrationOffset>32768</CalibrationOffset>\n      <CalibrationSlope>-65.8</CalibrationSlope>\n      <ParameterType>7</ParameterType>\n      <Description>Prefilter 1</Description>\n      <Linked>Equation</Linked>\n      <Unlinked>Operator</Unlinked>\n      <Location>Compound</Location>\n    </ParaRow>\n    <ParaRow Row=\"15\">\n      <Parameter>Q1</Parameter>\n      <Channal>6</Channal>\n      <UserMin>0</UserMin>\n      <UserMax>10</UserMax>\n      <UserDefault>4.5</UserDefault>\n      <CalibrationOffset>32755</CalibrationOffset>\n      <CalibrationSlope>-131.3</CalibrationSlope>\n      <ParameterType>11</ParameterType>\n      <Description>Quadrupole 1</Description>\n      <Linked>Equation</Linked>\n      <Unlinked>Equation</Unlinked>\n      <Location>Resolution</Location>\n    </ParaRow>\n    <ParaRow Row=\"16\">\n      <Parameter>CC L1</Parameter>\n      <Channal>13</Channal>\n      <UserMin>-10</UserMin>\n      <UserMax>100</UserMax>\n      <UserDefault>10</UserDefault>\n      <CalibrationOffset>32768</CalibrationOffset>\n      <CalibrationSlope>-65.8</CalibrationSlope>\n      <ParameterType>7</ParameterType>\n      <Description>Collision Cell Lens 1</Description>\n      <Linked>Equation</Linked>\n      <Unlinked>Operator</Unlinked>\n      <Location>Compound</Location>\n    </ParaRow>\n    <ParaRow Row=\"17\">\n      <Parameter>CC L2</Parameter>\n      <Channal>14</Channal>\n      <UserMin>0</UserMin>\n      <UserMax>400</UserMax>\n      <UserDefault>100</UserDefault>\n      <CalibrationOffset>32768</CalibrationOffset>\n      <CalibrationSlope>-65.8</CalibrationSlope>\n      <ParameterType>7</ParameterType>\n      <Description>Collision Cell Lens 2</Description>\n      <Linked>Operator</Linked>\n      <Unlinked>Operator</Unlinked>\n      <Location>Compound</Location>\n    </ParaRow>\n    <ParaRow Row=\"18\">\n      <Parameter>CC</Parameter>\n      <Channal>23</Channal>\n      <UserMin>0</UserMin>\n      <UserMax>150</UserMax>\n      <UserDefault>50</UserDefault>\n      <CalibrationOffset>32768</CalibrationOffset>\n      <CalibrationSlope>-65.8</CalibrationSlope>\n      <ParameterType>7</ParameterType>\n      <Description>Collision Energy</Description>\n      <Linked>Operator</Linked>\n      <Unlinked>Operator</Unlinked>\n      <Location>Compound</Location>\n    </ParaRow>\n    <ParaRow Row=\"19\">\n      <Parameter>CC AF</Parameter>\n      <Channal>10</Channal>\n      <UserMin>-400</UserMin>\n      <UserMax>0</UserMax>\n      <UserDefault>-100</UserDefault>\n      <CalibrationOffset>32768</CalibrationOffset>\n      <CalibrationSlope>-65.8</CalibrationSlope>\n      <ParameterType>7</ParameterType>\n      <Description>Axial Field</Description>\n      <Linked>Fixed</Linked>\n      <Unlinked>Operator</Unlinked>\n      <Location>Compound</Location>\n    </ParaRow>\n    <ParaRow Row=\"20\">\n      <Parameter>CC L3</Parameter>\n      <Channal>15</Channal>\n      <UserMin>0</UserMin>\n      <UserMax>200</UserMax>\n      <UserDefault>51</UserDefault>\n      <CalibrationOffset>32768</CalibrationOffset>\n      <CalibrationSlope>-65.7</CalibrationSlope>\n      <ParameterType>7</ParameterType>\n      <Description>Collision Cell Lens 3</Description>\n      <Linked>Equation</Linked>\n      <Unlinked>Equation</Unlinked>\n      <Location>Compound</Location>\n    </ParaRow>\n    <ParaRow Row=\"21\">\n      <Parameter>CC L4</Parameter>\n      <Channal>16</Channal>\n      <UserMin>0</UserMin>\n      <UserMax>400</UserMax>\n      <UserDefault>62</UserDefault>\n      <CalibrationOffset>32768</CalibrationOffset>\n      <CalibrationSlope>-65.7</CalibrationSlope>\n      <ParameterType>7</ParameterType>\n      <Description>Collision Cell Lens 4</Description>\n      <Linked>Equation</Linked>\n      <Unlinked>Equation</Unlinked>\n      <Location>Compound</Location>\n    </ParaRow>\n    <ParaRow Row=\"22\">\n      <Parameter>Q2</Parameter>\n      <Channal>8</Channal>\n      <UserMin>0</UserMin>\n      <UserMax>150</UserMax>\n      <UserDefault>52</UserDefault>\n      <CalibrationOffset>32756</CalibrationOffset>\n      <CalibrationSlope>-131.3</CalibrationSlope>\n      <ParameterType>11</ParameterType>\n      <Description>Quadrupole 2</Description>\n      <Linked>Equation</Linked>\n      <Unlinked>Equation</Unlinked>\n      <Location>Resolution</Location>\n    </ParaRow>\n    <ParaRow Row=\"23\">\n      <Parameter>ID</Parameter>\n      <Channal>17</Channal>\n      <UserMin>0</UserMin>\n      <UserMax>400</UserMax>\n      <UserDefault>160</UserDefault>\n      <CalibrationOffset>32768</CalibrationOffset>\n      <CalibrationSlope>-65.8</CalibrationSlope>\n      <ParameterType>7</ParameterType>\n      <Description>Detector Deflector</Description>\n      <Linked>Equation</Linked>\n      <Unlinked>Operator</Unlinked>\n      <Location>Compound</Location>\n    </ParaRow>\n    <ParaRow Row=\"24\">\n      <Parameter>DISC</Parameter>\n      <Channal>32</Channal>\n      <UserMin>10</UserMin>\n      <UserMax>2000</UserMax>\n      <UserDefault>15</UserDefault>\n      <CalibrationOffset>-5</CalibrationOffset>\n      <CalibrationSlope>1.23</CalibrationSlope>\n      <ParameterType>18</ParameterType>\n      <Description>Discriminator</Description>\n      <Linked>Fixed</Linked>\n      <Unlinked>Fixed</Unlinked>\n      <Location>Detector</Location>\n    </ParaRow>\n    <ParaRow Row=\"25\">\n      <Parameter>DV</Parameter>\n      <Channal>34</Channal>\n      <UserMin>1600</UserMin>\n      <UserMax>3500</UserMax>\n      <UserDefault>2000</UserDefault>\n      <CalibrationOffset>0</CalibrationOffset>\n      <CalibrationSlope>0.415</CalibrationSlope>\n      <ParameterType>18</ParameterType>\n      <Description>Detector Voltage</Description>\n      <Linked>Operator</Linked>\n      <Unlinked>Operator</Unlinked>\n      <Location>Detector</Location>\n    </ParaRow>\n    <ParaRow Row=\"26\">\n      <Parameter>DET horn</Parameter>\n      <Channal>200</Channal>\n      <UserMin>0</UserMin>\n      <UserMax>5500</UserMax>\n      <UserDefault>5500</UserDefault>\n      <CalibrationOffset>0</CalibrationOffset>\n      <CalibrationSlope>0.415</CalibrationSlope>\n      <ParameterType>16</ParameterType>\n      <Description>Detector Horn</Description>\n      <Linked>Fixed</Linked>\n      <Unlinked>Fixed</Unlinked>\n      <Location>Detector</Location>\n    </ParaRow>\n    <ParaRow Row=\"27\">\n      <Parameter>LS400A</Parameter>\n      <Channal>36</Channal>\n      <UserMin>0</UserMin>\n      <UserMax>420</UserMax>\n      <UserDefault>420</UserDefault>\n      <CalibrationOffset>0</CalibrationOffset>\n      <CalibrationSlope>8.4</CalibrationSlope>\n      <ParameterType>64</ParameterType>\n      <Description>Lens Power Supply A +400</Description>\n      <Linked>\n      </Linked>\n      <Unlinked>\n      </Unlinked>\n      <Location>\n      </Location>\n    </ParaRow>\n    <ParaRow Row=\"28\">\n      <Parameter>LS-400A</Parameter>\n      <Channal>37</Channal>\n      <UserMin>-420</UserMin>\n      <UserMax>-55</UserMax>\n      <UserDefault>-420</UserDefault>\n      <CalibrationOffset>-433</CalibrationOffset>\n      <CalibrationSlope>-8.4</CalibrationSlope>\n      <ParameterType>64</ParameterType>\n      <Description>Lens Power Supply A -400</Description>\n      <Linked>\n      </Linked>\n      <Unlinked>\n      </Unlinked>\n      <Location>\n      </Location>\n    </ParaRow>\n    <ParaRow Row=\"29\">\n      <Parameter>LS400B</Parameter>\n      <Channal>38</Channal>\n      <UserMin>0</UserMin>\n      <UserMax>420</UserMax>\n      <UserDefault>420</UserDefault>\n      <CalibrationOffset>0</CalibrationOffset>\n      <CalibrationSlope>8.4</CalibrationSlope>\n      <ParameterType>64</ParameterType>\n      <Description>Lens Power Supply B +400</Description>\n      <Linked>\n      </Linked>\n      <Unlinked>\n      </Unlinked>\n      <Location>\n      </Location>\n    </ParaRow>\n    <ParaRow Row=\"30\">\n      <Parameter>LS-400B</Parameter>\n      <Channal>39</Channal>\n      <UserMin>-420</UserMin>\n      <UserMax>-55</UserMax>\n      <UserDefault>-420</UserDefault>\n      <CalibrationOffset>-433</CalibrationOffset>\n      <CalibrationSlope>-8.4</CalibrationSlope>\n      <ParameterType>64</ParameterType>\n      <Description>Lens Power Supply B  -400</Description>\n      <Linked>\n      </Linked>\n      <Unlinked>\n      </Unlinked>\n      <Location>\n      </Location>\n    </ParaRow>\n    <ParaRow Row=\"31\">\n      <Parameter>QPS800</Parameter>\n      <Channal>40</Channal>\n      <UserMin>110</UserMin>\n      <UserMax>600</UserMax>\n      <UserDefault>600</UserDefault>\n      <CalibrationOffset>0</CalibrationOffset>\n      <CalibrationSlope>4.25</CalibrationSlope>\n      <ParameterType>64</ParameterType>\n      <Description>Quad Power Supply +800</Description>\n      <Linked>\n      </Linked>\n      <Unlinked>\n      </Unlinked>\n      <Location>\n      </Location>\n    </ParaRow>\n    <ParaRow Row=\"32\">\n      <Parameter>QPS-800</Parameter>\n      <Channal>41</Channal>\n      <UserMin>-110</UserMin>\n      <UserMax>-110</UserMax>\n      <UserDefault>-600</UserDefault>\n      <CalibrationOffset>-433</CalibrationOffset>\n      <CalibrationSlope>-4.2</CalibrationSlope>\n      <ParameterType>64</ParameterType>\n      <Description>Quad Power Supply -800</Description>\n      <Linked>\n      </Linked>\n      <Unlinked>\n      </Unlinked>\n      <Location>\n      </Location>\n    </ParaRow>\n    <ParaRow Row=\"33\">\n      <Parameter>DG</Parameter>\n      <Channal>26</Channal>\n      <UserMin>50</UserMin>\n      <UserMax>300</UserMax>\n      <UserDefault>80</UserDefault>\n      <CalibrationOffset>0</CalibrationOffset>\n      <CalibrationSlope>32.765</CalibrationSlope>\n      <ParameterType>32</ParameterType>\n      <Description>Drying Gas</Description>\n      <Linked>Operator</Linked>\n      <Unlinked>Operator</Unlinked>\n      <Location>Source</Location>\n    </ParaRow>\n    <ParaRow Row=\"34\">\n      <Parameter>NG1</Parameter>\n      <Channal>27</Channal>\n      <UserMin>0</UserMin>\n      <UserMax>450</UserMax>\n      <UserDefault>0</UserDefault>\n      <CalibrationOffset>0</CalibrationOffset>\n      <CalibrationSlope>32.765</CalibrationSlope>\n      <ParameterType>32</ParameterType>\n      <Description>Nebulizer Gas 1</Description>\n      <Linked>Operator</Linked>\n      <Unlinked>Operator</Unlinked>\n      <Location>Source</Location>\n    </ParaRow>\n    <ParaRow Row=\"35\">\n      <Parameter>HG1</Parameter>\n      <Channal>29</Channal>\n      <UserMin>0</UserMin>\n      <UserMax>350</UserMax>\n      <UserDefault>0</UserDefault>\n      <CalibrationOffset>0</CalibrationOffset>\n      <CalibrationSlope>32.765</CalibrationSlope>\n      <ParameterType>32</ParameterType>\n      <Description>Heating Gas 1</Description>\n      <Linked>Equation</Linked>\n      <Unlinked>Equation</Unlinked>\n      <Location>Source</Location>\n    </ParaRow>\n    <ParaRow Row=\"36\">\n      <Parameter>NG2</Parameter>\n      <Channal>28</Channal>\n      <UserMin>0</UserMin>\n      <UserMax>450</UserMax>\n      <UserDefault>0</UserDefault>\n      <CalibrationOffset>0</CalibrationOffset>\n      <CalibrationSlope>32.765</CalibrationSlope>\n      <ParameterType>32</ParameterType>\n      <Description>Nebulizer Gas 2</Description>\n      <Linked>Operator</Linked>\n      <Unlinked>Operator</Unlinked>\n      <Location>Source</Location>\n    </ParaRow>\n    <ParaRow Row=\"37\">\n      <Parameter>HG2</Parameter>\n      <Channal>30</Channal>\n      <UserMin>0</UserMin>\n      <UserMax>350</UserMax>\n      <UserDefault>0</UserDefault>\n      <CalibrationOffset>0</CalibrationOffset>\n      <CalibrationSlope>32.765</CalibrationSlope>\n      <ParameterType>32</ParameterType>\n      <Description>Heating Gas 2</Description>\n      <Linked>Equation</Linked>\n      <Unlinked>Equation</Unlinked>\n      <Location>Source</Location>\n    </ParaRow>\n    <ParaRow Row=\"38\">\n      <Parameter>CC P</Parameter>\n      <Channal>43</Channal>\n      <UserMin>0</UserMin>\n      <UserMax>500</UserMax>\n      <UserDefault>410</UserDefault>\n      <CalibrationOffset>0</CalibrationOffset>\n      <CalibrationSlope>32.765</CalibrationSlope>\n      <ParameterType>6</ParameterType>\n      <Description>Collision Pressure</Description>\n      <Linked>Fixed</Linked>\n      <Unlinked>Operator</Unlinked>\n      <Location>Compound</Location>\n    </ParaRow>\n    <ParaRow Row=\"39\">\n      <Parameter>SX</Parameter>\n      <Channal>42</Channal>\n      <UserMin>0</UserMin>\n      <UserMax>500</UserMax>\n      <UserDefault>500</UserDefault>\n      <CalibrationOffset>0</CalibrationOffset>\n      <CalibrationSlope>32.765</CalibrationSlope>\n      <ParameterType>32</ParameterType>\n      <Description>Source Exhaust</Description>\n      <Linked>Fixed</Linked>\n      <Unlinked>Fixed</Unlinked>\n      <Location>Source</Location>\n    </ParaRow>\n    <ParaRow Row=\"40\">\n      <Parameter>ISV2</Parameter>\n      <Channal>204</Channal>\n      <UserMin>-5850</UserMin>\n      <UserMax>0</UserMax>\n      <UserDefault>0</UserDefault>\n      <CalibrationOffset>0</CalibrationOffset>\n      <CalibrationSlope>0.0436</CalibrationSlope>\n      <ParameterType>34</ParameterType>\n      <Description>ElectroSpray V2</Description>\n      <Linked>Operator</Linked>\n      <Unlinked>Operator</Unlinked>\n      <Location>Source</Location>\n    </ParaRow>\n    <ParaRow Row=\"41\">\n      <Parameter>ISV1</Parameter>\n      <Channal>203</Channal>\n      <UserMin>-5850</UserMin>\n      <UserMax>0</UserMax>\n      <UserDefault>0</UserDefault>\n      <CalibrationOffset>0</CalibrationOffset>\n      <CalibrationSlope>0.0436</CalibrationSlope>\n      <ParameterType>34</ParameterType>\n      <Description>ElectroSpray V1</Description>\n      <Linked>Operator</Linked>\n      <Unlinked>Operator</Unlinked>\n      <Location>Source</Location>\n    </ParaRow>\n    <ParaRow Row=\"42\">\n      <Parameter>CD</Parameter>\n      <Channal>202</Channal>\n      <UserMin>-5</UserMin>\n      <UserMax>0</UserMax>\n      <UserDefault>0</UserDefault>\n      <CalibrationOffset>0</CalibrationOffset>\n      <CalibrationSlope>51</CalibrationSlope>\n      <ParameterType>34</ParameterType>\n      <Description>Corona Discharge</Description>\n      <Linked>Operator</Linked>\n      <Unlinked>Operator</Unlinked>\n      <Location>Source</Location>\n    </ParaRow>\n    <ParaRow Row=\"43\">\n      <Parameter>CAP</Parameter>\n      <Channal>201</Channal>\n      <UserMin>-1100</UserMin>\n      <UserMax>0</UserMax>\n      <UserDefault>-1000</UserDefault>\n      <CalibrationOffset>0</CalibrationOffset>\n      <CalibrationSlope>0.22</CalibrationSlope>\n      <ParameterType>34</ParameterType>\n      <Description>Curtain Cap</Description>\n      <Linked>Fixed</Linked>\n      <Unlinked>Fixed</Unlinked>\n      <Location>Source</Location>\n    </ParaRow>\n    <ParaRow Row=\"44\">\n      <Parameter>HSID T</Parameter>\n      <Channal>81</Channal>\n      <UserMin>0</UserMin>\n      <UserMax>320</UserMax>\n      <UserDefault>200</UserDefault>\n      <CalibrationOffset>0</CalibrationOffset>\n      <CalibrationSlope>1</CalibrationSlope>\n      <ParameterType>32</ParameterType>\n      <Description>HSID Temperature</Description>\n      <Linked>Operator</Linked>\n      <Unlinked>Operator</Unlinked>\n      <Location>Source</Location>\n    </ParaRow>\n    <ParaRow Row=\"45\">\n      <Parameter>P1 T</Parameter>\n      <Channal>86</Channal>\n      <UserMin>0</UserMin>\n      <UserMax>500</UserMax>\n      <UserDefault>0</UserDefault>\n      <CalibrationOffset>0</CalibrationOffset>\n      <CalibrationSlope>1</CalibrationSlope>\n      <ParameterType>32</ParameterType>\n      <Description>Source 1 Temp</Description>\n      <Linked>Operator</Linked>\n      <Unlinked>Operator</Unlinked>\n      <Location>Source</Location>\n    </ParaRow>\n    <ParaRow Row=\"46\">\n      <Parameter>P2 T</Parameter>\n      <Channal>84</Channal>\n      <UserMin>0</UserMin>\n      <UserMax>500</UserMax>\n      <UserDefault>0</UserDefault>\n      <CalibrationOffset>0</CalibrationOffset>\n      <CalibrationSlope>1</CalibrationSlope>\n      <ParameterType>32</ParameterType>\n      <Description>Source 2 Temp</Description>\n      <Linked>Operator</Linked>\n      <Unlinked>Operator</Unlinked>\n      <Location>Source</Location>\n    </ParaRow>\n  </ScanType>"]
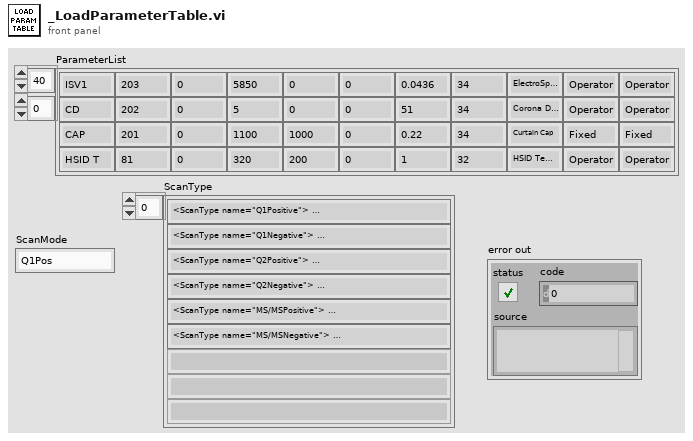
[diagram p1: front panel]
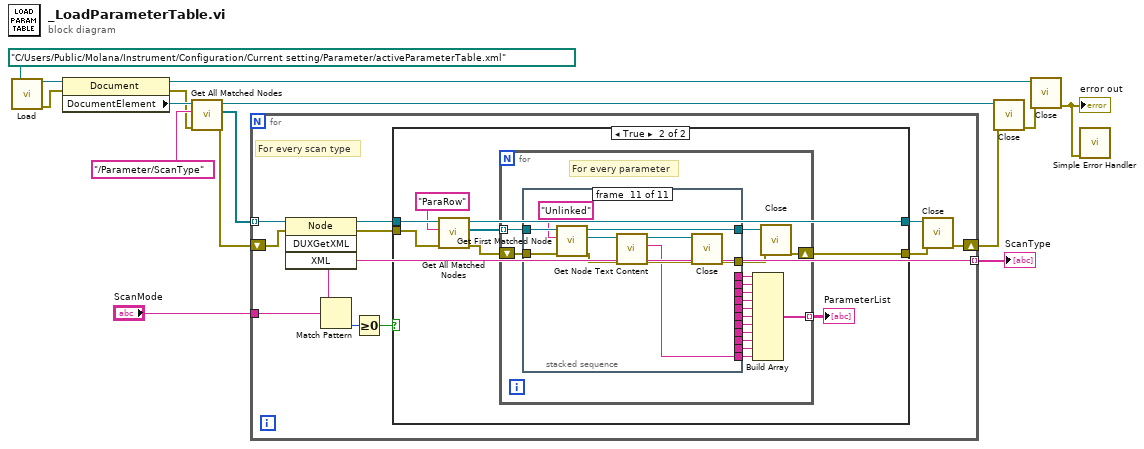
[diagram p0: block diagram]
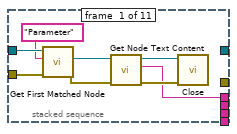
[diagram p3: hidden frame]
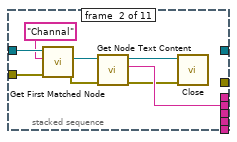
[diagram p4: hidden frame]
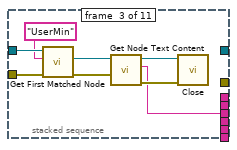
[diagram p5: hidden frame]
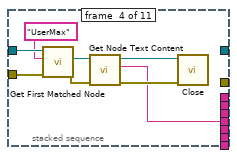
[diagram p6: hidden frame]
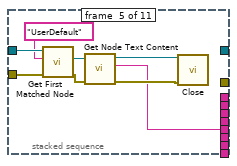
[diagram p7: hidden frame]
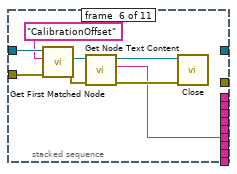
[diagram p8: hidden frame]
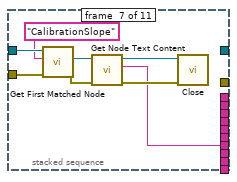
[diagram p9: hidden frame]
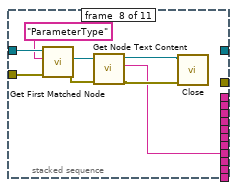
[diagram p10: hidden frame]
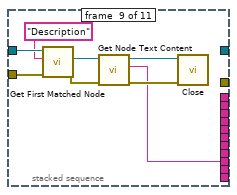
[diagram p11: hidden frame]
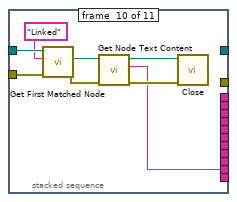
[diagram p12: hidden frame]
diagram:
  n1 = call-poly <vilib>:"Load.vi"("path to XML document"=path "C:/Users/Public/Molana/Instrument/Configuration/Current setting/Parameter/activeParameterTable.xml" ("Path")) -> ("DOM document out"=w15:refnum<k20>, "error out"=w14:errorcluster)  [unwired: 12 in, 1 out]
  n2 = property on="Property Node" class="Document"(reference=w15, error in=w14) -> (reference out=w11:refnum<k20>, error out=w6:errorcluster, "DocumentElement"=w7:refnum<k20>)
  n3 = call <vilib>:"Get All Matched Nodes.vi"("error in (no error)"=w6, "XPath expression"="/Parameter/ScanType", "node in"=w7) -> ("error out"=w4:errorcluster, "node result array"=w8:refnum<k20>[], "node out"=w5:refnum<k20>)  [unwired: 6 in]
  n4 = for {
    tunnel: w8 -> [w26] mode=indexing
    shift-right: [w17] -> w3
    shift-left: w4 -> [w25]
    tunnel: [w20] -> w2 mode=indexing
    tunnel: "ScanMode" -> [w16]
    # "For every scan type"
    n5 = invoke on="Invoke Node" class="Node" method="DUXGetXML"(reference=w26, error in=w25) -> (reference out=w22:refnum<k20>, error out=w21:errorcluster, "XML"=w20:string)  [unwired: 2 in, 1 out]
    n6 = Match Pattern(string=w20, regular expression=w16) -> (offset past match=w19:i32)  [unwired: 1 in, 3 out]
    n7 = Greater Or Equal To 0?(x=w19) -> (x >= 0?=w18:bool)
    n8 = case shown="True" w18 {
      tunnel: [w27 w30] -> w24
      tunnel: [w28 w33] -> w23
      tunnel: w22 -> [w28 w36]
      tunnel: w21 -> [w27 w35]
      frame False {
      }
      frame True {
        n9 = call <vilib>:"Get All Matched Nodes.vi"("error in (no error)"=w35, "XPath expression"="ParaRow" ("regular expression"), "node in"=w36) -> ("error out"=w31:errorcluster, "node result array"=w32:refnum<k20>[], "node out"=w33:refnum<k20>)  [unwired: 6 in]
        n10 = for {
          tunnel: w32 -> [w42] mode=indexing
          shift-right: [w40] -> w30
          shift-left: w31 -> [w41]
          tunnel: [w37] -> w29 mode=indexing
          # "For every parameter"
          n11 = stacked-sequence {
            tunnel: w42 -> [w61 w69 w77 w85 w93 w101 w109 w117 w125 w133 w143]
            tunnel: w41 -> [w60 w68 w76 w84 w92 w100 w108 w116 w124 w132 w142]
            tunnel: [w54 _ _ _ _ _ _ _ _ _ _] -> w43
            tunnel: [_ w65 _ _ _ _ _ _ _ _ _] -> w44
            tunnel: [_ _ w70 _ _ _ _ _ _ _ _] -> w45
            tunnel: [_ _ _ w78 _ _ _ _ _ _ _] -> w46
            tunnel: [_ _ _ _ w86 _ _ _ _ _ _] -> w47
            tunnel: [_ _ _ _ _ w94 _ _ _ _ _] -> w48
            tunnel: [_ _ _ _ _ _ w102 _ _ _ _] -> w49
            tunnel: [_ _ _ _ _ _ _ w110 _ _ _] -> w50
            tunnel: [_ _ _ _ _ _ _ _ w118 _ _] -> w51
            tunnel: [_ _ _ _ _ _ _ _ _ _ w140] -> w39
            tunnel: [_ _ _ _ _ _ _ _ _ _ w139] -> w38
            tunnel: [_ _ _ _ _ _ _ _ _ _ w134] -> w52
            tunnel: [_ _ _ _ _ _ _ _ _ w126 _] -> w53
            frame #0 {
              n12 = call <vilib>:"Get First Matched Node.vi"("error in (no error)"=w60, "XPath expression"="Parameter", "node in"=w61) -> ("error out"=w57:errorcluster, "node result"=w58:refnum<k20>)  [unwired: 6 in, 1 out]
              n13 = call <vilib>:"Get Node Text Content.vi"("error in (no error)"=w57, "node in"=w58) -> ("error out"=w55:errorcluster, "node text"=w54:string, "node out"=w56:refnum<k20>)  [unwired: 7 in]
              n14 = call-poly <vilib>:"Close.vi"("error in (no error)"=w55, "node"=w56) -> ()  [unwired: 7 in, 1 out]
            }
            frame #1 {
              n15 = call <vilib>:"Get First Matched Node.vi"("error in (no error)"=w68, "XPath expression"="Channal", "node in"=w69) -> ("error out"=w62:errorcluster, "node result"=w66:refnum<k20>)  [unwired: 6 in, 1 out]
              n16 = call <vilib>:"Get Node Text Content.vi"("error in (no error)"=w62, "node in"=w66) -> ("error out"=w63:errorcluster, "node text"=w65:string, "node out"=w64:refnum<k20>)  [unwired: 7 in]
              n17 = call-poly <vilib>:"Close.vi"("error in (no error)"=w63, "node"=w64) -> ()  [unwired: 7 in, 1 out]
            }
            frame #2 {
              n18 = call <vilib>:"Get First Matched Node.vi"("error in (no error)"=w76, "XPath expression"="UserMin", "node in"=w77) -> ("error out"=w73:errorcluster, "node result"=w74:refnum<k20>)  [unwired: 6 in, 1 out]
              n19 = call <vilib>:"Get Node Text Content.vi"("error in (no error)"=w73, "node in"=w74) -> ("error out"=w72:errorcluster, "node text"=w70:string, "node out"=w71:refnum<k20>)  [unwired: 7 in]
              n20 = call-poly <vilib>:"Close.vi"("error in (no error)"=w72, "node"=w71) -> ()  [unwired: 7 in, 1 out]
            }
            frame #3 {
              n21 = call <vilib>:"Get First Matched Node.vi"("error in (no error)"=w84, "XPath expression"="UserMax", "node in"=w85) -> ("error out"=w81:errorcluster, "node result"=w82:refnum<k20>)  [unwired: 6 in, 1 out]
              n22 = call <vilib>:"Get Node Text Content.vi"("error in (no error)"=w81, "node in"=w82) -> ("error out"=w79:errorcluster, "node text"=w78:string, "node out"=w80:refnum<k20>)  [unwired: 7 in]
              n23 = call-poly <vilib>:"Close.vi"("error in (no error)"=w79, "node"=w80) -> ()  [unwired: 7 in, 1 out]
            }
            frame #4 {
              n24 = call <vilib>:"Get First Matched Node.vi"("error in (no error)"=w92, "XPath expression"="UserDefault", "node in"=w93) -> ("error out"=w88:errorcluster, "node result"=w90:refnum<k20>)  [unwired: 6 in, 1 out]
              n25 = call <vilib>:"Get Node Text Content.vi"("error in (no error)"=w88, "node in"=w90) -> ("error out"=w87:errorcluster, "node text"=w86:string, "node out"=w89:refnum<k20>)  [unwired: 7 in]
              n26 = call-poly <vilib>:"Close.vi"("error in (no error)"=w87, "node"=w89) -> ()  [unwired: 7 in, 1 out]
            }
            frame #5 {
              n27 = call <vilib>:"Get First Matched Node.vi"("error in (no error)"=w100, "XPath expression"="CalibrationOffset", "node in"=w101) -> ("error out"=w96:errorcluster, "node result"=w98:refnum<k20>)  [unwired: 6 in, 1 out]
              n28 = call <vilib>:"Get Node Text Content.vi"("error in (no error)"=w96, "node in"=w98) -> ("error out"=w95:errorcluster, "node text"=w94:string, "node out"=w97:refnum<k20>)  [unwired: 7 in]
              n29 = call-poly <vilib>:"Close.vi"("error in (no error)"=w95, "node"=w97) -> ()  [unwired: 7 in, 1 out]
            }
            frame #6 {
              n30 = call <vilib>:"Get First Matched Node.vi"("error in (no error)"=w108, "XPath expression"="CalibrationSlope", "node in"=w109) -> ("error out"=w105:errorcluster, "node result"=w106:refnum<k20>)  [unwired: 6 in, 1 out]
              n31 = call <vilib>:"Get Node Text Content.vi"("error in (no error)"=w105, "node in"=w106) -> ("error out"=w104:errorcluster, "node text"=w102:string, "node out"=w103:refnum<k20>)  [unwired: 7 in]
              n32 = call-poly <vilib>:"Close.vi"("error in (no error)"=w104, "node"=w103) -> ()  [unwired: 7 in, 1 out]
            }
            frame #7 {
              n33 = call <vilib>:"Get First Matched Node.vi"("error in (no error)"=w116, "XPath expression"="ParameterType", "node in"=w117) -> ("error out"=w113:errorcluster, "node result"=w114:refnum<k20>)  [unwired: 6 in, 1 out]
              n34 = call <vilib>:"Get Node Text Content.vi"("error in (no error)"=w113, "node in"=w114) -> ("error out"=w111:errorcluster, "node text"=w110:string, "node out"=w112:refnum<k20>)  [unwired: 7 in]
              n35 = call-poly <vilib>:"Close.vi"("error in (no error)"=w111, "node"=w112) -> ()  [unwired: 7 in, 1 out]
            }
            frame #8 {
              n36 = call <vilib>:"Get First Matched Node.vi"("error in (no error)"=w124, "XPath expression"="Description", "node in"=w125) -> ("error out"=w119:errorcluster, "node result"=w122:refnum<k20>)  [unwired: 6 in, 1 out]
              n37 = call <vilib>:"Get Node Text Content.vi"("error in (no error)"=w119, "node in"=w122) -> ("error out"=w120:errorcluster, "node text"=w118:string, "node out"=w121:refnum<k20>)  [unwired: 7 in]
              n38 = call-poly <vilib>:"Close.vi"("error in (no error)"=w120, "node"=w121) -> ()  [unwired: 7 in, 1 out]
            }
            frame #9 {
              n39 = call <vilib>:"Get First Matched Node.vi"("error in (no error)"=w132, "XPath expression"="Linked", "node in"=w133) -> ("error out"=w127:errorcluster, "node result"=w130:refnum<k20>)  [unwired: 6 in, 1 out]
              n40 = call <vilib>:"Get Node Text Content.vi"("error in (no error)"=w127, "node in"=w130) -> ("error out"=w128:errorcluster, "node text"=w126:string, "node out"=w129:refnum<k20>)  [unwired: 7 in]
              n41 = call-poly <vilib>:"Close.vi"("error in (no error)"=w128, "node"=w129) -> ()  [unwired: 7 in, 1 out]
            }
            frame #10 {
              n42 = call <vilib>:"Get First Matched Node.vi"("error in (no error)"=w142, "XPath expression"="Unlinked", "node in"=w143) -> ("error out"=w137:errorcluster, "node result"=w138:refnum<k20>, "node out"=w140:refnum<k20>)  [unwired: 6 in]
              n43 = call <vilib>:"Get Node Text Content.vi"("error in (no error)"=w137, "node in"=w138) -> ("error out"=w135:errorcluster, "node text"=w134:string, "node out"=w136:refnum<k20>)  [unwired: 7 in]
              n44 = call-poly <vilib>:"Close.vi"("error in (no error)"=w135, "node"=w136) -> ("error out"=w139:errorcluster)  [unwired: 7 in]
            }
          }
          n45 = Build Array(w43, w44, w45, w46, w47, w48, w49, w50, w51, w53, w52) -> (w37:string[])
          n46 = call-poly <vilib>:"Close.vi"("error in (no error)"=w38, "node"=w39) -> ("error out"=w40:errorcluster)  [unwired: 7 in]
        }
        "ParameterList" <- w29
      }
    }
    n47 = call-poly <vilib>:"Close.vi"("error in (no error)"=w24, "node"=w23) -> ("error out"=w17:errorcluster)  [unwired: 7 in]
  }
  "ScanType" <- w2
  n48 = call-poly <vilib>:"Close.vi"("error in (no error)"=w3, "node"=w5) -> ("error out"=w10:errorcluster)  [unwired: 7 in]
  n49 = call-poly <vilib>:"Close.vi"("error in (no error)"=w10, "node"=w11) -> ("error out"=w9:errorcluster)  [unwired: 7 in]
  "error out" <- w9
  n50 = call <vilib>:"Simple Error Handler.vi"("error in (no error)"=w9) -> ()  [unwired: 4 in, 5 out]
